vi "BStAT_(Doubles) Update.vi"() -> ()   [LabVIEW 2013]
uses:
  <vilib>/vision/Image Controls.llb/IMAQ Image.ctl
  <vilib>/Utility/file.llb/Read From Spreadsheet File (string).vi
  <vilib>/Utility/file.llb/Read From Spreadsheet File (I64).vi
panel:
  in  "fast rewind":bool
  out "refnum of data save file":refnum<file>
  in  "START":bool
  out "frames to write":i64[][](array[numeric])
  in  "Data file":path caption="Data"
  in  "playback speed":dbl(slide)=1.0 min=0.25 max=1.5 step=0.25 scale=0.25..1.5
  in  "Main tab":enum32{"Coding", "Display"}(tab)
  in  "9 6":bool
  in  "10 6":bool
  in  "9 5":bool
  in  "10 5":bool
  in  "10 3":bool
  in  "9 3":bool
  in  "10 4":bool
  in  "9 4":bool
  in  "9 2":bool
  in  "10 2":bool
  in  "10":bool
  in  "9":bool
  in  "1 6":bool
  in  "2 6":bool
  in  "3 6":bool
  in  "4 6":bool
  in  "5 6":bool
  in  "6 6":bool
  in  "7 6":bool
  in  "8 6":bool
  in  "1 5":bool
  in  "2 5":bool
  in  "3 5":bool
  in  "4 5":bool
  in  "5 5":bool
  in  "6 5":bool
  in  "7 5":bool
  in  "8 5":bool
  in  "8 3":bool
  in  "7 3":bool
  in  "6 3":bool
  in  "5 3":bool
  in  "4 3":bool
  in  "3 3":bool
  in  "2 3":bool
  in  "1 3":bool
  in  "8 4":bool
  in  "7 4":bool
  in  "6 4":bool
  in  "5 4":bool
  in  "4 4":bool
  in  "3 4":bool
  in  "2 4":bool
  in  "1 4":bool
  in  "1 2":bool
  in  "2 2":bool
  in  "3 2":bool
  in  "4 2":bool
  in  "5 2":bool
  in  "6 2":bool
  in  "7 2":bool
  in  "8 2":bool
  in  "5":bool
  in  "6":bool
  in  "7":bool
  in  "8":bool
  in  "1":bool
  in  "2":bool
  in  "3":bool
  in  "4":bool
  in  "Player 3":bool
  in  "Player 4":bool
  in  "MCL 3":bool
  in  "BCL 3":bool
  in  "TCL 3":bool
  in  "TCR 2":bool
  in  "MCR 2":bool
  in  "BCR 2":bool
  in  "TCR 3":bool
  in  "MCR  3":bool
  in  "BCR 3":bool
  in  "MCL 2":bool
  in  "BCL 2":bool
  in  "TCL 2":bool
  in  "Player 2":bool
  in  "Player 1":bool
  in  "TC 3":bool
  in  "TR 3":bool
  in  "ML 3":bool
  in  "MC 3":bool
  in  "MR  3":bool
  in  "BC 3":bool
  in  "BL 3":bool
  in  "BR 3":bool
  in  "TL 3":bool
  in  "TC 2":bool
  in  "TR 2":bool
  in  "ML 2":bool
  in  "MC 2":bool
  in  "MR  2":bool
  in  "BC 2":bool
  in  "BL 2":bool
  in  "BR 2":bool
  in  "TL 2":bool
  in  "Name 4":string
  in  "Name 3":string
  in  "Name 2":string
  in  "Name 1":string
  in  "5 7":bool
  in  "S3":bool
  in  "S4":bool
  in  "Switch position":bool
  in  "Link Errors":bool
  in  "E2":bool
  in  "E1":bool
  in  "W2":bool
  in  "W1":bool
  in  "P2":i32
  in  "P1":i32
  in  "S1":bool
  in  "S2":bool
  in  "1 7":bool
  in  "2 7":bool
  in  "3 7":bool
  in  "4 7":bool
  in  "Code lag(s)":dbl=1.0 min=0.0 max=5.0 step=0.5 format="%#.1g"
  in  "Pause lag(s)":dbl=1.0 min=0.0 max=2.0 step=0.5 format="%#.1g"
  in  "Pause lag on":bool
  in  "Display tab":enum32{"Edit ", "Data Display", "Momentum"}(tab)
  in  "player4":bool
  in  "player3":bool
  in  "player1":bool
  in  "player2":bool
  in  "Team 1":bool
  in  "Team 2":bool
  in  "service4":bool
  in  "service3":bool
  in  "5 8":bool
  in  "1 9":bool
  in  "service2":bool
  in  "service1":bool
  in  "2 9":bool
  in  "3 8":bool
  in  "4 8":bool
  in  "Blk def":bool
  in  "clear def":bool
  in  "lob":bool
  in  "clear":bool
  in  "drive":bool
  in  "smash":bool
  in  "Dr def":bool
  in  "Hf smash":bool
  in  "drop":bool
  in  "net":bool
  in  "FH 2":bool
  in  "BH 2":bool
  in  "ST":bool
  in  "CR 2":bool
  in  "OH 2":bool
  in  "BCR":bool
  in  "MCR":bool
  in  "TCR":bool
  in  "TCL":bool
  in  "BCL":bool
  in  "MCL":bool
  in  "TL":bool
  in  "BR":bool
  in  "BL":bool
  in  "BC":bool
  in  "MR":bool
  in  "MC":bool
  in  "ML":bool
  in  "TR":bool
  in  "TC":bool
  in  "REPORT":bool
  out "Video files to write":string[](array[string])
  in  "Video compress":bool=TRUE
  in  "Abort":bool
  in  "Write file":bool
  in  "Delete":bool[](array[boolean])
  out "Writing":u32(slide) scale=0.0..51.0
  in  "File name":string
  in  "Add to lib":bool
  in  "Video to write":path caption="Folder"
  in  "Examine code":bool
  in  "Update":bool
  in  "Reset":bool
  out "Code number display":i32
  in  "Next":bool
  in  "Previous":bool
  in  "after":u8(slide)=2 scale=0.0..5.0
  in  "before":u8(slide)=2
  in  "point 2":bool
  in  "error":bool
  in  "winner":bool
  in  "point 1":bool
  in  "Extract data":bool
  in  "Upload edited video":bool
  in  "To make white":enum32{""}(tab)
  out "player1 2":string[](array[string])=["0", "0", "0", "0", "0", "0", "0", "0", "0", "0"]
  out "player2 2":string[](array[string])=["0", "0", "0", "0", "0", "0", "0", "0", "0", "0"]
  out "p2 23":string
  out "p2 22":string
  out "p2 21":string
  out "p2 20":string
  out "p2 19":string
  out "p2 18":string
  out "p1 15":string
  out "p1 14":string
  out "p1 13":string
  out "p1 12":string
  out "p1 11":string
  out "p1 10":string
  out "p2 17":string
  out "p2 16":string
  out "p2 11":string
  out "p2 10":string
  out "p2 9":string
  out "p2 14":string
  out "p2 13":string
  out "p2 12":string
  out "p2 15":string
  out "p1 5":string
  out "p1 7":string
  out "p1 6":string
  out "p1 4":string
  out "p1 1":string
  out "p1 3":string
  out "p1 2":string
  out "p1 8":string
  out "p1 9":string
  out "Player 5":string[](array[string])=["Fore hand", "Back hand", "Over head", "", "Straight", "Cross", "", "Smash", "Half smash", "DRIVE DEF", "BLOCK DEF", "CLEAR DEF", "Drive/Tap", "Lob", "Drop", "Clear", "Net"]
  out "Player 6":string[](array[string])=["Fore hand", "Back hand", "Over head", "", "Straight", "Cross", "", "Smash", "Half smash", "DRIVE DEF", "BLOCK DEF", "CLEAR DEF", "Drive/Tap", "Lob", "Drop", "Clear", "Net"]
  out "player1_2":string[](array[string])=["0", "0", "0", "", "0", "0"]
  out "W2/E2":string[](array[string])=["0", "0"]
  out "Player 2_2":string[](array[string])=["Fore hand", "Back hand", "Over head", "", "Strainght", "Cross", "", "Lob", "Clear", "Drive", "Smash", "Defence", "Chop", "Drop", "Net"]
  out "W/E2":string[](array[string])=["Fore hand", "Back hand", "Over head", "", "Strainght", "Cross", "", "Lob", "Clear", "Drive", "Smash", "Defence", "Chop", "Drop", "Net"]
  out "player2_2":string[](array[string])=["0", "0", "0", "", "0", "0"]
  out "W1/E1":string[](array[string])=["0", "0"]
  out "Player 1_2":string[](array[string])=["Fore hand", "Back hand", "Over head", "", "Strainght", "Cross", "", "Lob", "Clear", "Drive", "Smash", "Defence", "Chop", "Drop", "Net"]
  out "W/E1":string[](array[string])=["Fore hand", "Back hand", "Over head", "", "Strainght", "Cross", "", "Lob", "Clear", "Drive", "Smash", "Defence", "Chop", "Drop", "Net"]
  out "P2graph":cluster{dbl[], "array":dbl[]}(graph)={[0.0, nan, 0.0, nan, 0.0, nan, 0.0, nan, 0.0, nan, 0.0, nan, 0.0, nan, 0.0, nan, 0.0], "array"=[1.0, 2.0, 3.0, 4.0, 5.0, 6.0, 7.0, 8.0, 9.0, 10.0, 11.0, 12.0, 13.0, 14.0, 15.0, 16.0, 17.0]}
  out "P1graph":cluster{dbl[], "array":dbl[]}(graph)={[0.0, nan, 0.0, nan, 0.0, nan, 0.0, nan, 0.0, nan, 0.0, nan, 0.0, nan, 0.0, nan, 0.0], "array"=[1.0, 2.0, 3.0, 4.0, 5.0, 6.0, 7.0, 8.0, 9.0, 10.0, 11.0, 12.0, 13.0, 14.0, 15.0, 16.0, 17.0]}
  in  "save2":string
  in  "save1":string
  in  "save2 3":bool
  in  "save1 3":bool
  in  "Compare":bool
  in  "2 8":string(combo)="1"
  in  "1 8":string(combo)="1"
  in  "display\nselection":string(combo)="1"
  in  "Percentage":bool
  in  "to make white 2":enum32{""}(tab)
  out "Shortest rally length(sec)":dbl format="%#_3g"
  out "Longest rally length(sec)":dbl format="%#_3g"
  out "Score":dbl[](array[numeric])
  out "Average rally length(sec)":dbl format="%#_3g"
  out "Rally length(sec)":dbl format="%#_3g"
  out "momentum graph":cluster{dbl[], dbl[]}[](graph)
  in  "Code number":i32 min=0 max=28
  in  "Load video":bool
  in  "Play":bool
  out "ful video frames":i64[](array[numeric])
  out "playback speed":dbl
  out "Number of Frames":u32
  out "framesPerSecond":u32
  out "Last Edit":bool[](array[boolean])
  out "frames 2 play":i64[](array[numeric])
  in  "stop":bool
  out "Video Frame":u32
  out "save1 2":i32[][](array[numeric])
  out "save1_data":dbl[][](array[numeric])
  out "save2 2":i32[][](array[numeric])
  out "save2_data":dbl[][](array[numeric])
  out "game":i32[][](array[numeric])
  out "comp_p1":dbl[](array[numeric])
  out "comp_p2":dbl[](array[numeric])
  out "comp_p2 2":dbl[](array[numeric])
  out "comp_p1 2":dbl[](array[numeric])
  out "Score 2":i64[][](array[numeric])
  out "frame data":i64[][](array[numeric])
  out "coded data":i64[][](array[numeric])
  out "edited\nevents":i64[][](array[numeric])
  out "edited to play":i64[](array[numeric])
  out "frames edited":i64[](array[numeric])
  out "service frames":i64[](array[numeric])
  out "point frames":i64[](array[numeric])
  out "p1y":dbl[](array[numeric])
  out "p2y":dbl[](array[numeric])
  in  "fast forward":bool
  in  "Pause":bool
  out "coding":i64[][](array[numeric])
  out "FH":bool[](array[boolean])
  out "BH":bool[](array[boolean])
  out "OH":bool[](array[boolean])
  out "P1 position":bool
  out "P2 position":bool
  in  "Progress...":u32(slide) min=400 max=47374 scale=-1.1..47174.0
  in  "Video file":path caption="Video"
  out "task":i32(slide) scale=0.0..300.0
  out "Video":T1(plugin-control)
  # "Strategic Analysis Tool for Badminton"
  # "© 2012 National Sports Institute of Malaysia All Rights Reserved"
  # "Position"
  # "Rally start"
  # "Rally end"
  # "Forehand"
  # "Backhand"
  # "Overhead"
  # "Straight"
  # "Cross"
  # "Straight"
  # "Cross"
  # "Straight"
  # "Cross"
  # "Smash"
  # "Half Smash"
  # "DRIVE Defence"
  # "BLOCK Defence"
  # "CLEAR Defence"
  # "Drive/Tap"
  # "Lob"
  # "Drop"
  # "Clear"
  # "Net"
  # "Switch sides"
  # "Player"
  # "Team"
  # "Rally start"
  # "Shots"
  # "Position"
  # "Playback interval (s)"
  # "Rally end"
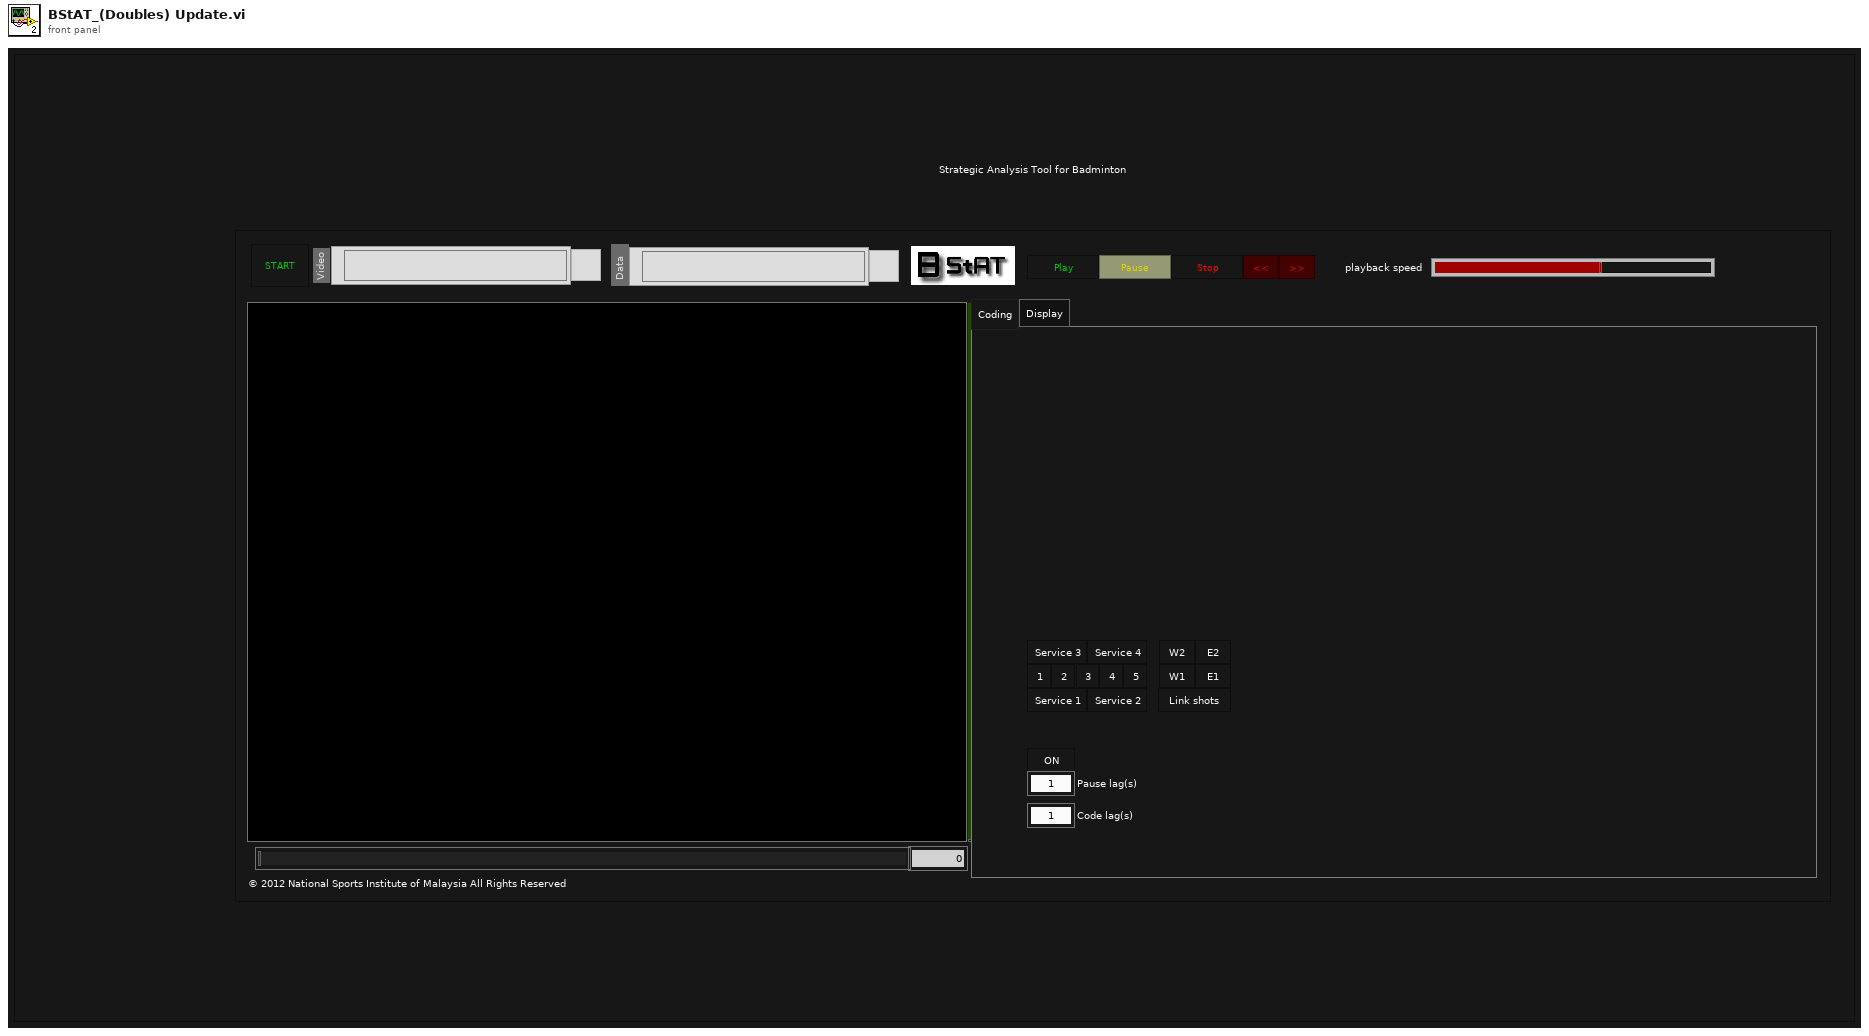
[diagram p1: front panel]
types:
  T1 = typedef "IMAQ Image.ctl" = refnum<image>
  T2 = enum32{"Coding", "Edit video", "Examine coding", "Display", "Update coding", "Edit coding"}
  T3 = enum16{"open", "replace", "create", "open or create", "replace or create", "replace or create with confirmation"}
  T4 = enum8{"Enabled", "Disabled", "Disabled and Grayed Out"}
  T5 = typedef "Image Type" = u32
  T6 = typedef "AviRefnum.ctl" = refnum<k1>
  T7 = cluster{"width":u32, "height":u32, "framesPerSecond":u32, "compressionFilter":string, "hasData":bool}
  T8 = typedef "LVPositionTypeDef.ctl" = cluster{"Left":i32, "Top":i32}
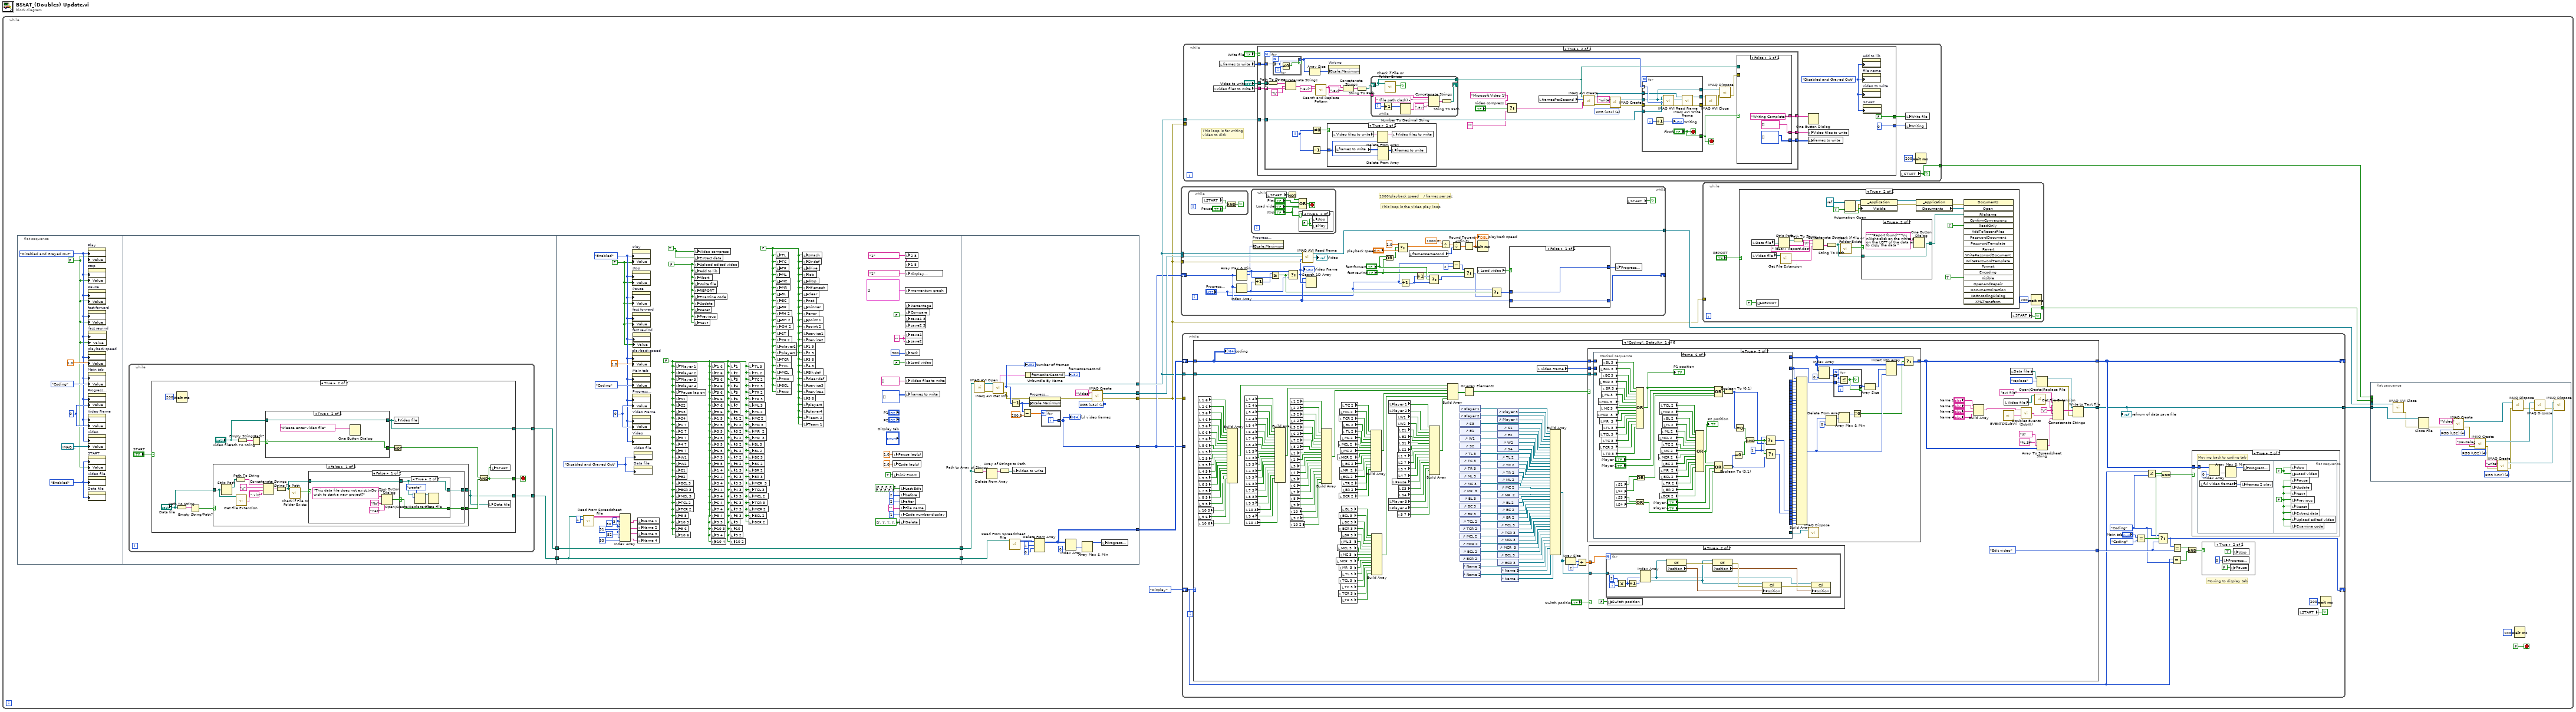
[diagram p0: block diagram]
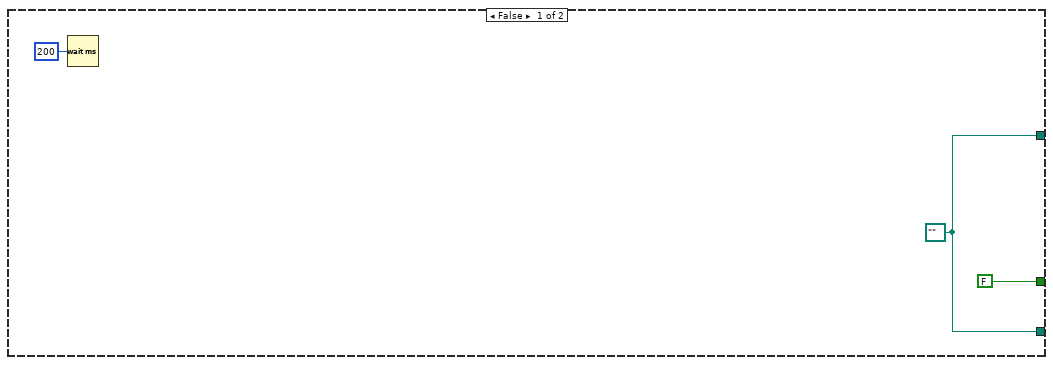
[diagram p2: hidden frame]
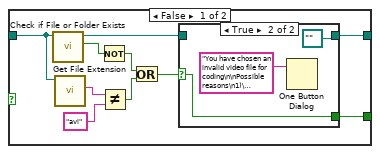
[diagram p3: hidden frame]
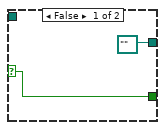
[diagram p5: hidden frame]
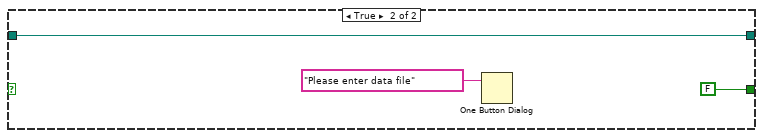
[diagram p7: hidden frame]
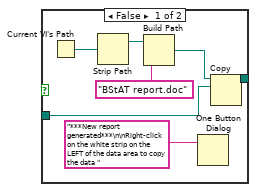
[diagram p9: hidden frame]
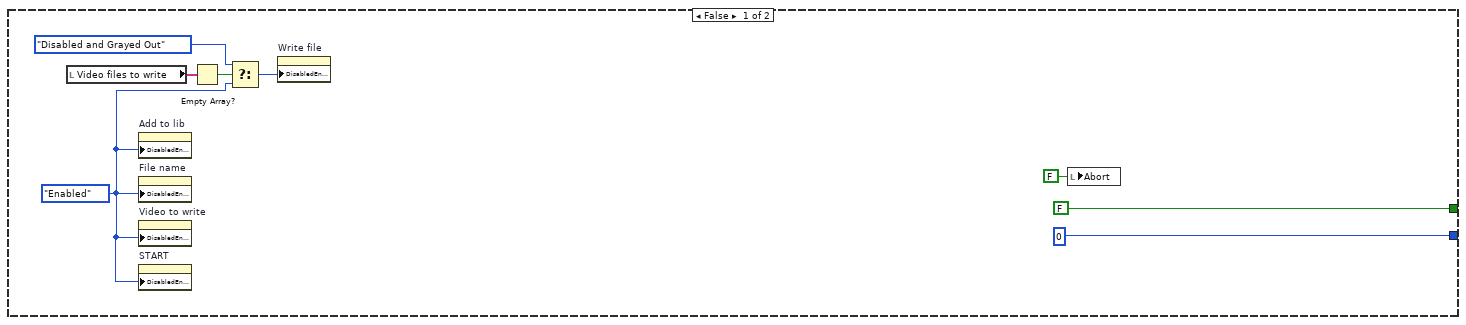
[diagram p10: hidden frame]
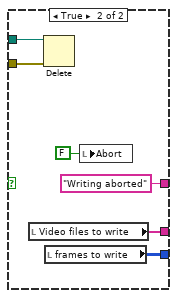
[diagram p11: hidden frame]
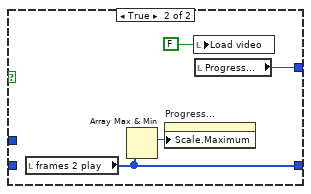
[diagram p14: hidden frame]
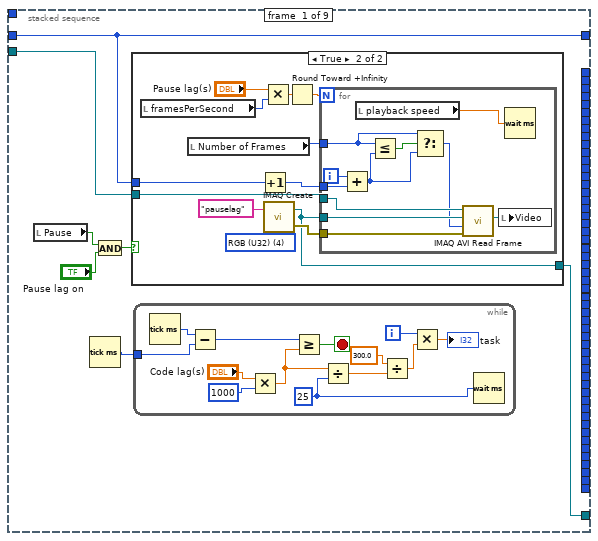
[diagram p19: hidden frame]
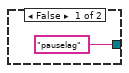
[diagram p20: hidden frame]
diagram:
  n1 = while {
    stop <- FALSE stop-if-true
    n2 = flat-sequence {
      tunnel: [w42] -> w15
      tunnel: [w43] -> w16
      tunnel: w16 -> [w152]
      tunnel: w15 -> [w133]
      tunnel: [w133] -> w14
      tunnel: [w152] -> w13
      tunnel: w14 -> [w174]
      tunnel: w13 -> [w157]
      tunnel: [w173] -> w11
      tunnel: [w156] -> w10
      tunnel: [w155] -> w9
      tunnel: [w154] -> w1
      tunnel: [w153] -> w8
      frame #0 {
        w37 = T4."Enabled" ("Disabled")
        w39 = u32 0 ("Progress...")
        w35 = FALSE ("START")
        w36 = T4."Disabled and Grayed Out" ("Disabled")
        n3 = property on="Play" class="Bool (strict)"("DisabledEnum"=w36, "Value"=w35) -> ()  [unwired: 2 in, 2 out]
        n4 = property on="stop" class="Bool (strict)"("DisabledEnum"=w36, "Value"=w35) -> ()  [unwired: 2 in, 2 out]
        n5 = property on="Pause" class="Bool (strict)"("DisabledEnum"=w36, "Value"=w35) -> ()  [unwired: 2 in, 2 out]
        n6 = property on="fast forward" class="Bool (strict)"("DisabledEnum"=w36, "Value"=w35) -> ()  [unwired: 2 in, 2 out]
        n7 = property on="playback speed" class="Slide (strict)"("DisabledEnum"=w36, "Value"=1.0 ("playback speed")) -> ()  [unwired: 2 in, 2 out]
        n8 = property on="Main tab" class="TabCtl (strict)"("DisabledEnum"=w36, "Value"=enum32{"Coding", "Display"}."Coding" ("Main tab")) -> ()  [unwired: 2 in, 2 out]
        n9 = property on="Progress..." class="Slide (strict)"("DisabledEnum"=w36, "Value"=w39) -> ()  [unwired: 2 in, 2 out]
        n10 = property on="Video Frame" class="DigNum (strict)"("DisabledEnum"=w36, "Value"=w39) -> ()  [unwired: 2 in, 2 out]
        n11 = property on="Video" class="ImageControl"("DisabledEnum"=w36, "Value"=T1 refnum ("Video")) -> ()  [unwired: 2 in, 2 out]
        n12 = property on="START" class="Bool (strict)"("DisabledEnum"=w37, "Value"=w35) -> ()  [unwired: 2 in, 2 out]
        n13 = property on="Video file" class="Path"("DisabledEnum"=w37) -> ()  [unwired: 2 in, 2 out]
        n14 = property on="Data file" class="Path"("DisabledEnum"=w37) -> ()  [unwired: 2 in, 2 out]
        n15 = property on="fast rewind" class="Bool (strict)"("DisabledEnum"=w36, "Value"=w35) -> ()  [unwired: 2 in, 2 out]
      }
      frame #1 {
        n16 = while {
          tunnel: [w45] -> w43
          tunnel: [w44] -> w42
          stop <- w46 stop-if-true
          n17 = case shown="True" "START" {
            tunnel: [FALSE w51] -> w46
            tunnel: [w48 w54] -> w45
            tunnel: [w48 w53] -> w44
            frame False {
              w48 = path "" ("dup path")
              n18 = Wait (ms)(milliseconds to wait=u32 200) -> ()  [unwired: 1 out]
            }
            frame True {
              n19 = Path To String(path="Data file") -> (string=w63:string)
              n20 = Wait (ms)(milliseconds to wait=u32 200) -> ()  [unwired: 1 out]
              n21 = Empty String/Path?(string/path=w63) -> (empty?=w62:bool)
              n22 = case shown="False" w62 {
                tunnel: "Data file" -> [w84 w109]
                tunnel: [w83 FALSE] -> w60
                tunnel: [w82 w109] -> w53
                frame False {
                  n23 = Strip Path(path=w84) -> (stripped path=w89:path)  [unwired: 1 out]
                  n24 = Path To String(path=w89) -> (string=w88:string)
                  n25 = call <vilib>:"Get File Extension.vi"("file"=w84) -> ("filename without extension"=w91:string)  [unwired: 7 in, 3 out]
                  n26 = Concatenate Strings(w88, "\\" ("string"), w91, ".xls" ("string")) -> (w90:string)
                  n27 = String To Path(string=w90) -> (path=w85:path)
                  n28 = call <vilib>:"Check if File or Folder Exists.vi"("path"=w85) -> ("file or folder exists?"=w86:bool)  [unwired: 8 in, 2 out]
                  n29 = case shown="False" w86 {
                    selector: w86 -> [_ w108]
                    tunnel: w85 -> [w95 w107]
                    tunnel: [w94 w108] -> w83
                    tunnel: [w93 w107] -> w82
                    frame False {
                      n30 = Two Button Dialog(message="This data file does not exist.\nDo you wish to start a new project?", 1:"No" ("F button name (\"Cancel\")"), 2:"Yes" ("T button name (\"OK\")")) -> (T button?=w96:bool)
                      n31 = case shown="True" w96 {
                        selector: w96 -> [w101 w103]
                        tunnel: w95 -> [_ w102]
                        tunnel: [w101 w103] -> w94
                        tunnel: [path "" ("dup path") w102] -> w93
                        frame False {
                        }
                        frame True {
                          n32 = Open/Create/Replace File(file path (use dialog)=w102, operation (0:open)=T3."create") -> (refnum out=w104:refnum<file>, error out=w106:errorcluster)  [unwired: 4 in, 1 out]
                          n33 = Close File(refnum=w104, error in=w106) -> ()  [unwired: 2 out]
                        }
                      }
                    }
                    frame True {
                    }
                  }
                }
                frame True {
                  n34 = One Button Dialog(message="Please enter data file") -> ()  [unwired: 1 in, 1 out]
                }
              }
              n35 = Path To String(path="Video file") -> (string=w58:string)
              n36 = Empty String/Path?(string/path=w58) -> (empty?=w57:bool)
              n37 = case shown="True" w57 {
                selector: w57 -> [_ w81]
                tunnel: "Video file" -> [w68 w79]
                tunnel: [w65 w79] -> w54
                tunnel: [w64 w81] -> w55
                frame False {
                  n38 = call <vilib>:"Check if File or Folder Exists.vi"("path"=w68) -> ("file or folder exists?"=w72:bool, "dup path"=w66:path)  [unwired: 8 in, 1 out]
                  n39 = call <vilib>:"Get File Extension.vi"("file"=w68) -> ("lowercase file extension"=w69:string)  [unwired: 7 in, 3 out]
                  n40 = Not(x=w72) -> (.not. x?=w73:bool)
                  n41 = Not Equal?(x=w69, y="avi" ("lowercase file extension")) -> (x != y?=w71:bool)
                  n42 = Or(x=w73, y=w71) -> (x .or. y?=w67:bool)
                  n43 = case shown="True" w67 {
                    selector: w67 -> [w74 w76]
                    tunnel: w66 -> [w75 _]
                    tunnel: [w75 path "" ("dup path")] -> w65
                    tunnel: [w74 w76] -> w64
                    frame False {
                    }
                    frame True {
                      n44 = One Button Dialog(message="You have chosen an invalid video file for coding\n\nPossible reasons\n1)\tChosen video file format was not AVI\n2)\tChosen video file does not exist") -> ()  [unwired: 1 in, 1 out]
                    }
                  }
                }
                frame True {
                  n45 = One Button Dialog(message="Please enter video file") -> ()  [unwired: 1 in, 1 out]
                }
              }
              n46 = Not(x=w55) -> (.not. x?=w59:bool)
              n47 = local write "Video file"(w54) -> ()
              n48 = And(x=w59, y=w60) -> (x .and. y?=w51:bool)
              n49 = local write "Data file"(w53) -> ()
              n50 = local write "START"(w51) -> ()
            }
          }
        }
      }
      frame #2 {
        w130 = 3 ("index (row)")
        w138 = "" ("save2")
        w139 = "1" ("2 8")
        w142 = FALSE ("4 6")
        w121 = FALSE ("4 6")
        w147 = FALSE ("4 6")
        w120 = FALSE ("4 6")
        w146 = TRUE ("Extract data")
        w148 = T4."Disabled and Grayed Out" ("Disabled")
        w151 = u32 0 ("Progress...")
        w112 = FALSE ("START")
        w113 = T4."Enabled" ("Disabled")
        n51 = call-poly <vilib>:"Read From Spreadsheet File.vi"("number of rows (all:-1)"=4, "file path (dialog if empty)"=w133) -> ("all rows"=w131:string[][])  [unwired: 5 in, 4 out]
        n52 = Index Array(array=w131, index (row) #1=w130, index (col) #1=50 ("disabled index (col)"), index (row) #2=w130, index (col) #2=51 ("disabled index (col)"), index (row) #3=w130, index (col) #3=52 ("disabled index (col)"), index (row) #4=w130, index (col) #4=53 ("disabled index (col)")) -> (element #1=w122:string, element #2=w125:string, element #3=w124:string, element #4=w123:string)
        n53 = property on="Play" class="Bool (strict)"("DisabledEnum"=w113, "Value"=w112) -> ()  [unwired: 2 in, 2 out]
        n54 = property on="stop" class="Bool (strict)"("DisabledEnum"=w113, "Value"=w112) -> ()  [unwired: 2 in, 2 out]
        n55 = property on="Pause" class="Bool (strict)"("DisabledEnum"=w113, "Value"=w112) -> ()  [unwired: 2 in, 2 out]
        n56 = property on="fast forward" class="Bool (strict)"("DisabledEnum"=w113, "Value"=w112) -> ()  [unwired: 2 in, 2 out]
        n57 = property on="playback speed" class="Slide (strict)"("DisabledEnum"=w113, "Value"=1.0 ("playback speed")) -> ()  [unwired: 2 in, 2 out]
        n58 = property on="Main tab" class="TabCtl (strict)"("DisabledEnum"=w113, "Value"=enum32{"Coding", "Display"}."Coding" ("Main tab")) -> ()  [unwired: 2 in, 2 out]
        n59 = property on="Progress..." class="Slide (strict)"("DisabledEnum"=w113, "Value"=w151) -> ()  [unwired: 2 in, 2 out]
        n60 = property on="Video Frame" class="DigNum (strict)"("DisabledEnum"=w113, "Value"=w151) -> ()  [unwired: 2 in, 2 out]
        n61 = property on="Video" class="ImageControl"("DisabledEnum"=w113) -> ()  [unwired: 2 in, 2 out]
        n62 = property on="fast rewind" class="Bool (strict)"("DisabledEnum"=w113, "Value"=w112) -> ()  [unwired: 2 in, 2 out]
        n63 = property on="Video file" class="Path"("DisabledEnum"=w148) -> ()  [unwired: 2 in, 2 out]
        n64 = property on="Data file" class="Path"("DisabledEnum"=w148) -> ()  [unwired: 2 in, 2 out]
        n65 = local write "Name 1"(w122) -> ()
        n66 = local write "Name 2"(w125) -> ()
        n67 = local write "Name 3"(w124) -> ()
        n68 = local write "Name 4"(w123) -> ()
        n69 = local write "Player 1"(w121) -> ()
        n70 = local write "Player 2"(w121) -> ()
        n71 = local write "Player 3"(w121) -> ()
        n72 = local write "Player 4"(w121) -> ()
        n73 = local write "Pause lag on"(w121) -> ()
        n74 = local write "S1"(w121) -> ()
        n75 = local write "S2"(w121) -> ()
        n76 = local write "S3"(w121) -> ()
        n77 = local write "S4"(w121) -> ()
        n78 = local write "1 7"(w121) -> ()
        n79 = local write "2 7"(w121) -> ()
        n80 = local write "3 7"(w121) -> ()
        n81 = local write "4 7"(w121) -> ()
        n82 = local write "5 7"(w121) -> ()
        n83 = local write "W1"(w121) -> ()
        n84 = local write "W2"(w121) -> ()
        n85 = local write "E1"(w121) -> ()
        n86 = local write "E2"(w121) -> ()
        n87 = local write "BCL 3"(w121) -> ()
        n88 = local write "BCR 3"(w121) -> ()
        n89 = local write "MCL 3"(w121) -> ()
        n90 = local write "TCL 2"(w121) -> ()
        n91 = local write "TCR 2"(w121) -> ()
        n92 = local write "9 5"(w121) -> ()
        n93 = local write "10 5"(w121) -> ()
        n94 = local write "9 6"(w121) -> ()
        n95 = local write "10 6"(w121) -> ()
        n96 = local write "Video compress"(w146) -> ()
        n97 = local write "Extract data"(w146) -> ()
        n98 = local write "Upload edited video"(w147) -> ()
        n99 = local write "Add to lib"(w147) -> ()
        n100 = local write "Abort"(w147) -> ()
        n101 = local write "Write file"(w147) -> ()
        n102 = local write "REPORT"(w147) -> ()
        n103 = local write "Examine code"(w147) -> ()
        n104 = local write "Update"(w147) -> ()
        n105 = local write "Reset"(w147) -> ()
        n106 = local write "Previous"(w147) -> ()
        n107 = local write "Next"(w147) -> ()
        n108 = local write "1 6"(w121) -> ()
        n109 = local write "2 6"(w121) -> ()
        n110 = local write "3 6"(w121) -> ()
        n111 = local write "4 6"(w121) -> ()
        n112 = local write "5 6"(w121) -> ()
        n113 = local write "6 6"(w121) -> ()
        n114 = local write "7 6"(w121) -> ()
        n115 = local write "8 6"(w121) -> ()
        n116 = local write "1 5"(w121) -> ()
        n117 = local write "2 5"(w121) -> ()
        n118 = local write "3 5"(w121) -> ()
        n119 = local write "4 5"(w121) -> ()
        n120 = local write "5 5"(w121) -> ()
        n121 = local write "6 5"(w121) -> ()
        n122 = local write "7 5"(w121) -> ()
        n123 = local write "8 5"(w121) -> ()
        n124 = local write "1 4"(w121) -> ()
        n125 = local write "2 4"(w121) -> ()
        n126 = local write "3 4"(w121) -> ()
        n127 = local write "4 4"(w121) -> ()
        n128 = local write "5 4"(w121) -> ()
        n129 = local write "6 4"(w121) -> ()
        n130 = local write "7 4"(w121) -> ()
        n131 = local write "8 4"(w121) -> ()
        n132 = local write "9 3"(w121) -> ()
        n133 = local write "10 3"(w121) -> ()
        n134 = local write "9 4"(w121) -> ()
        n135 = local write "10 4"(w121) -> ()
        n136 = local write "1"(w121) -> ()
        n137 = local write "2"(w121) -> ()
        n138 = local write "3"(w121) -> ()
        n139 = local write "4"(w121) -> ()
        n140 = local write "5"(w121) -> ()
        n141 = local write "6"(w121) -> ()
        n142 = local write "7"(w121) -> ()
        n143 = local write "8"(w121) -> ()
        n144 = local write "1 2"(w121) -> ()
        n145 = local write "2 2"(w121) -> ()
        n146 = local write "3 2"(w121) -> ()
        n147 = local write "4 2"(w121) -> ()
        n148 = local write "5 2"(w121) -> ()
        n149 = local write "6 2"(w121) -> ()
        n150 = local write "7 2"(w121) -> ()
        n151 = local write "8 2"(w121) -> ()
        n152 = local write "1 3"(w121) -> ()
        n153 = local write "2 3"(w121) -> ()
        n154 = local write "3 3"(w121) -> ()
        n155 = local write "4 3"(w121) -> ()
        n156 = local write "5 3"(w121) -> ()
        n157 = local write "6 3"(w121) -> ()
        n158 = local write "7 3"(w121) -> ()
        n159 = local write "8 3"(w121) -> ()
        n160 = local write "9"(w121) -> ()
        n161 = local write "10"(w121) -> ()
        n162 = local write "9 2"(w121) -> ()
        n163 = local write "10 2"(w121) -> ()
        n164 = local write "TL 3"(w121) -> ()
        n165 = local write "TL 2"(w121) -> ()
        n166 = local write "TC 2"(w121) -> ()
        n167 = local write "TC 3"(w121) -> ()
        n168 = local write "TR 2"(w121) -> ()
        n169 = local write "TR 3"(w121) -> ()
        n170 = local write "ML 3"(w121) -> ()
        n171 = local write "ML 2"(w121) -> ()
        n172 = local write "MC 2"(w121) -> ()
        n173 = local write "MC 3"(w121) -> ()
        n174 = local write "MR  2"(w121) -> ()
        n175 = local write "MR  3"(w121) -> ()
        n176 = local write "BL 3"(w121) -> ()
        n177 = local write "BL 2"(w121) -> ()
        n178 = local write "BC 3"(w121) -> ()
        n179 = local write "BC 2"(w121) -> ()
        n180 = local write "BR 2"(w121) -> ()
        n181 = local write "BR 3"(w121) -> ()
        n182 = local write "MCR  3"(w121) -> ()
        n183 = local write "TCL 3"(w121) -> ()
        n184 = local write "MCL 2"(w121) -> ()
        n185 = local write "TCR 3"(w121) -> ()
        n186 = local write "MCR 2"(w121) -> ()
        n187 = local write "BCL 2"(w121) -> ()
        n188 = local write "BCR 2"(w121) -> ()
        n189 = local write "TL"(w120) -> ()
        n190 = local write "TC"(w120) -> ()
        n191 = local write "TR"(w120) -> ()
        n192 = local write "ML"(w120) -> ()
        n193 = local write "MC"(w120) -> ()
        n194 = local write "MR"(w120) -> ()
        n195 = local write "BL"(w120) -> ()
        n196 = local write "BC"(w120) -> ()
        n197 = local write "BR"(w120) -> ()
        n198 = local write "FH 2"(w120) -> ()
        n199 = local write "BH 2"(w120) -> ()
        n200 = local write "OH 2"(w120) -> ()
        n201 = local write "ST"(w120) -> ()
        n202 = local write "CR 2"(w120) -> ()
        n203 = local write "player1"(w120) -> ()
        n204 = local write "player2"(w120) -> ()
        n205 = local write "TCR"(w120) -> ()
        n206 = local write "TCL"(w120) -> ()
        n207 = local write "MCL"(w120) -> ()
        n208 = local write "MCR"(w120) -> ()
        n209 = local write "BCL"(w120) -> ()
        n210 = local write "BCR"(w120) -> ()
        n211 = local write "smash"(w120) -> ()
        n212 = local write "Dr def"(w120) -> ()
        n213 = local write "drive"(w120) -> ()
        n214 = local write "lob"(w120) -> ()
        n215 = local write "drop"(w120) -> ()
        n216 = local write "Hf smash"(w120) -> ()
        n217 = local write "clear"(w120) -> ()
        n218 = local write "net"(w120) -> ()
        n219 = local write "winner"(w120) -> ()
        n220 = local write "error"(w120) -> ()
        n221 = local write "point 1"(w120) -> ()
        n222 = local write "point 2"(w120) -> ()
        n223 = local write "service1"(w120) -> ()
        n224 = local write "service2"(w120) -> ()
        n225 = local write "1 9"(w120) -> ()
        n226 = local write "2 9"(w120) -> ()
        n227 = local write "3 8"(w120) -> ()
        n228 = local write "4 8"(w120) -> ()
        n229 = local write "Blk def"(w120) -> ()
        n230 = local write "clear def"(w120) -> ()
        n231 = local write "service3"(w120) -> ()
        n232 = local write "service4"(w120) -> ()
        n233 = local write "5 8"(w120) -> ()
        n234 = local write "player3"(w120) -> ()
        n235 = local write "player4"(w120) -> ()
        n236 = local write "Team 2"(w120) -> ()
        n237 = local write "Team 1"(w120) -> ()
        n238 = local write "Pause lag(s)"(1.0 ("Pause lag(s)")) -> ()
        n239 = local write "Code lag(s)"(2.0 ("Code lag(s)")) -> ()
        n240 = local write "Link Errors"(TRUE ("Link Errors")) -> ()
        n241 = local write "Last Edit"(bool[] [FALSE, FALSE, FALSE, FALSE, FALSE, FALSE, FALSE, FALSE, FALSE, FALSE, FALSE, FALSE, FALSE, FALSE, FALSE, FALSE, FALSE, FALSE, FALSE, FALSE, FALSE, FALSE, FALSE, FALSE, FALSE, FALSE, FALSE, FALSE, FALSE, FALSE, FALSE, FALSE, FALSE, FALSE, FALSE, FALSE] ("Last Edit")) -> ()
        n242 = local write "before"(u8 2 ("before")) -> ()
        n243 = local write "after"(u8 2 ("after")) -> ()
        n244 = local write "File name"("" ("File name")) -> ()
        n245 = local write "Code number display"(1 ("Code number display")) -> ()
        n246 = local write "Delete"(bool[] [TRUE, TRUE, TRUE, TRUE, TRUE] ("Array 2")) -> ()
        n247 = local write "2 8"(w139) -> ()
        n248 = local write "1 8"(w139) -> ()
        n249 = local write "display\nselection"("1" ("display\nselection")) -> ()
        n250 = local write "momentum graph"(cluster{dbl[], dbl[]}[] [] ("momentum graph")) -> ()
        n251 = local write "Percentage"(w142) -> ()
        n252 = local write "Compare"(w142) -> ()
        n253 = local write "save1 3"(w142) -> ()
        n254 = local write "save2 3"(w142) -> ()
        n255 = local write "save1"(w138) -> ()
        n256 = local write "save2"(w138) -> ()
        n257 = local write "task"(300 ("task")) -> ()
        n258 = local write "Load video"(FALSE ("Pause")) -> ()
        n259 = local write "Video files to write"(string[] [] ("Video files to write")) -> ()
        n260 = local write "frames to write"(i64[][] [] ("to write")) -> ()
      }
      frame #3 {
        w159 = T5 4 items=["Grayscale (U8)", "Grayscale (I16)", "Grayscale (SGL)", "Complex (CSG)", "RGB (U32)", "HSL (U32)", "RGB (U64)"] ("Image Type")
        n261 = Path to Array of Strings(0:w157) -> (2:w170:string[])  [unwired: 1 out]
        n262 = call "IMAQ AVI Open"("AVI Path"=w157) -> ("error out"=w161:errorcluster, "Avi Refnum"=w160:T6)  [unwired: 9 in]
        n263 = Delete From Array(array=w170) -> (array with subset deleted=w171:string[])  [unwired: 2 in, 1 out]
        n264 = call "IMAQ AVI Get Info"("error in (no error)"=w161, "Avi Refnum"=w160) -> ("error out"=w163:errorcluster, "Number of Frames"=w166:u32, "Avi Refnum (duplicate)"=w156:T6, "Frame Data"=w162:T7)  [unwired: 5 in, 1 out]
        "Number of Frames" <- w166
        n265 = Array of Strings to Path(0:w171) -> (2:w172:path)  [unwired: 1 in]
        n266 = call-poly <vilib>:"Read From Spreadsheet File.vi"("file path (dialog if empty)"=w174) -> ("all rows"=w177:i64[][])  [unwired: 6 in, 4 out]
        n267 = Decrement(x=w166) -> (x-1=w169:u32)
        n268 = local write "Video to write"(w172) -> ()
        n269 = Subtract(x=w169, y=200.0) -> (x-y=w167:dbl)
        n270 = Unbundle By Name(w162) -> ("framesPerSecond"=→"framesPerSecond":u32)
        n271 = property on="Progress..." class="Slide (strict)"(error in=w163, "Scale.Maximum"=w169) -> (error out=w164:errorcluster)  [unwired: 1 in, 1 out]
        n272 = Delete From Array(array=w177, length=4, index (row)=0) -> (array with subset deleted=w173:i64[][])  [unwired: 1 in, 1 out]
        n273 = for {
          N: w167 -> [_]
          tunnel: [w181] -> w153 mode=indexing
          i -> [w181]
        }
        "ful video frames" <- w153
        n274 = Index Array(array=w173, index (col)=0 ("disabled index (col)")) -> (element=w179:i64[])  [unwired: 1 in]
        n275 = Array Max & Min(array=w179) -> (max value=w178:i64)  [unwired: 3 out]
        n276 = call "IMAQ Create"("Image Name"="Video", "Image Type"=w159, "error in (no error)"=w164) -> ("New Image"=w155:T1, "error out"=w154:errorcluster)  [unwired: 2 in]
        n277 = local write "Progress..."(w178) -> ()
      }
    }
    n278 = while {
      tunnel: w10 -> [w353]
      tunnel: w9 -> [w352]
      tunnel: w1 -> [w351]
      shift-right: [w345] -> _
      shift-left: w8 -> [w344]
      tunnel: [w329] -> w4
      stop <- w330 continue-if-true
      # "This loop is the video play loop"
      # "1000/playback speed    / frames per sec"
      n279 = while {
        stop <- w369 continue-if-true
        n280 = local read "START"() -> (w368:bool)
        n281 = And(x=w368, y="Pause") -> (x .and. y?=w369:bool)
      }
      n282 = Index Array(array=w344, index="Progress...") -> (element=w331:i64)
      n283 = Array Max & Min(array=w344) -> (max value=w349:i64, max index (indices)=w350:i32)  [unwired: 2 out]
      n284 = while {
        stop <- w358 stop-if-true
        n285 = local read "START"() -> (w355:bool)
        n286 = Not(x=w355) -> (.not. x?=w354:bool)
        n287 = Compound Arithmetic op=OR(w354, "Play", "Load video", "stop") -> (w358:bool)
        n288 = case shown="True" "stop" {
          frame False {
          }
          frame True {
            w360 = FALSE ("Play")
            n289 = local write "stop"(w360) -> ()
            n290 = local write "Play"(w360) -> ()
          }
        }
      }
      n291 = property on="Progress..." class="Slide (strict)"("Scale.Maximum"=w350) -> ()  [unwired: 2 in, 2 out]
      n292 = Increment(x=w331) -> (x+1=w332:i64)
      n293 = Greater Or Equal?(x=w332, y=w349) -> (x >= y?=w335:bool)
      n294 = Select(t=w349, s=w335, f=w331) -> (s? t:f=w346:i64)
      "Video Frame" <- w346
      n295 = call "IMAQ AVI Read Frame"("error in (no error)"=w351, "Frame Number"=w346, "Image"=w352, "Avi Refnum"=w353) -> ("Image Out"=→"Video":T1, "Avi Refnum (duplicate)"=w329:T6)  [unwired: 4 in, 2 out]
      n296 = Search 1D Array(1D array=w344, element=w346) -> ()  [unwired: 1 in, 1 out]
      n297 = Or(x="fast forward", y="fast rewind") -> (x .or. y?=w323:bool)
      n298 = Select(t=1.0, s=w323, f="playback speed") -> (s? t:f=w338:dbl)
      n299 = Increment(x="Progress...") -> (x+1=w325:u32)
      n300 = local read "framesPerSecond"() -> (w343:u32)
      n301 = Increment(x=w325) -> (x+1=w324:u32)
      n302 = Select(t=w324, s="fast forward", f=w325) -> (s? t:f=w327:u32)
      n303 = Divide(x=1000.0, y=w338) -> (x/y=w342:dbl)
      n304 = Subtract(x="Progress...", y=2) -> (x-y=w326:u32)
      n305 = Divide(x=w342, y=w343) -> (x/y=w340:dbl)
      n306 = Round Toward -Infinity(1:w340) -> (0:w339:dbl)
      "playback speed" <- w339
      n307 = Select(t=w326, s="fast rewind", f=w327) -> (s? t:f=w322:u32)
      n308 = Wait (ms)(milliseconds to wait=w339) -> ()  [unwired: 1 out]
      n309 = local read "Load video"() -> (w333:bool)
      n310 = Select(t="Progress...", s=w335, f=w322) -> (s? t:f=w334:u32)
      n311 = case shown="False" w333 {
        tunnel: w344 -> [w361 _]
        tunnel: w334 -> [w362 _]
        tunnel: [w362 w363] -> w348
        tunnel: [w361 w366] -> w345
        frame False {
        }
        frame True {
          n312 = local read "frames 2 play"() -> (w366:i64[])
          n313 = Array Max & Min(array=w366) -> (max index (indices)=w365:i32)  [unwired: 3 out]
          n314 = property on="Progress..." class="Slide (strict)"("Scale.Maximum"=w365) -> ()  [unwired: 2 in, 2 out]
          n315 = local write "Load video"(FALSE ("Play")) -> ()
          n316 = local read "Progress..."() -> (w363:u32)
        }
      }
      n317 = local write "Progress..."(w348) -> ()
      n318 = local read "START"() -> (w330:bool)
    }
    n319 = while {
      shift-right: [w379] -> _
      shift-left: T2."Display" ("Main tab") -> [w376]
      tunnel: w10 -> [w384]
      shift-right: [w372] -> _
      shift-left: w11 -> [w387]
      tunnel: w8 -> [_]
      tunnel: w1 -> [_]
      tunnel: [w370] -> w7
      stop <- w371 continue-if-true
      w375 = T2."Coding" ("Main tab")
      # "Moving to display tab"
      n320 = case shown="\"Coding\", Default" w376 {
        tunnel: w387 -> [w590 w1079 w1624 w1841 w1881 w1986]
        tunnel: [w511 w1079 w1624 w1841 w1881 w1972] -> w372
        tunnel: [T2."Edit video" ("Main tab") w1082 T2."Display" ("Main tab") T2."Edit coding" ("Main tab") w1882 T2."Edit video" ("Main tab")] -> w378
        tunnel: w384 -> [w523 _ _ _ _ _]
        tunnel: [w506 w1073 w1675 w1839 w1879 w1970] -> w370
        frame "Coding", Default {
          w517 = "\r"
          n321 = local read "1 6"() -> (w573:bool)
          n322 = local read "2 6"() -> (w574:bool)
          n323 = local read "3 6"() -> (w575:bool)
          n324 = local read "4 6"() -> (w576:bool)
          n325 = local read "5 6"() -> (w577:bool)
          n326 = local read "6 6"() -> (w578:bool)
          n327 = local read "7 6"() -> (w580:bool)
          n328 = local read "8 6"() -> (w579:bool)
          n329 = local read "1 5"() -> (w581:bool)
          n330 = local read "2 5"() -> (w582:bool)
          n331 = local read "3 5"() -> (w583:bool)
          n332 = local read "4 5"() -> (w584:bool)
          n333 = local read "5 5"() -> (w585:bool)
          n334 = local read "6 5"() -> (w586:bool)
          n335 = local read "7 5"() -> (w587:bool)
          n336 = local read "8 5"() -> (w588:bool)
          n337 = local read "9 5"() -> (w490:bool)
          n338 = local read "10 5"() -> (w489:bool)
          n339 = local read "9 6"() -> (w488:bool)
          n340 = local read "10 6"() -> (w487:bool)
          n341 = Build Array(w573, w574, w575, w576, w577, w578, w580, w579, w581, w582, w583, w584, w585, w586, w587, w588, w490, w489, w488, w487) -> (w521:bool[])
          n342 = local read "1 4"() -> (w557:bool)
          n343 = local read "2 4"() -> (w558:bool)
          n344 = local read "3 4"() -> (w559:bool)
          n345 = local read "4 4"() -> (w560:bool)
          n346 = local read "5 4"() -> (w561:bool)
          n347 = local read "6 4"() -> (w562:bool)
          n348 = local read "7 4"() -> (w563:bool)
          n349 = local read "8 4"() -> (w564:bool)
          n350 = local read "1 3"() -> (w565:bool)
          n351 = local read "2 3"() -> (w566:bool)
          n352 = local read "3 3"() -> (w567:bool)
          n353 = local read "4 3"() -> (w568:bool)
          n354 = local read "5 3"() -> (w569:bool)
          n355 = local read "6 3"() -> (w570:bool)
          n356 = local read "7 3"() -> (w571:bool)
          n357 = local read "8 3"() -> (w572:bool)
          n358 = local read "9 3"() -> (w494:bool)
          n359 = local read "10 3"() -> (w493:bool)
          n360 = local read "9 4"() -> (w492:bool)
          n361 = local read "10 4"() -> (w491:bool)
          n362 = Build Array(w557, w558, w559, w560, w561, w562, w563, w564, w565, w566, w567, w568, w569, w570, w571, w572, w494, w493, w492, w491) -> (w520:bool[])
          n363 = local read "1 2"() -> (w541:bool)
          n364 = local read "2 2"() -> (w542:bool)
          n365 = local read "3 2"() -> (w543:bool)
          n366 = local read "4 2"() -> (w544:bool)
          n367 = local read "5 2"() -> (w545:bool)
          n368 = local read "6 2"() -> (w546:bool)
          n369 = local read "7 2"() -> (w547:bool)
          n370 = local read "8 2"() -> (w548:bool)
          n371 = local read "1"() -> (w549:bool)
          n372 = local read "2"() -> (w550:bool)
          n373 = local read "3"() -> (w551:bool)
          n374 = local read "4"() -> (w552:bool)
          n375 = local read "5"() -> (w553:bool)
          n376 = local read "6"() -> (w554:bool)
          n377 = local read "7"() -> (w555:bool)
          n378 = local read "8"() -> (w556:bool)
          n379 = local read "9"() -> (w498:bool)
          n380 = local read "10"() -> (w497:bool)
          n381 = local read "9 2"() -> (w496:bool)
          n382 = local read "10 2"() -> (w495:bool)
          n383 = Build Array(w541, w542, w543, w544, w545, w546, w547, w548, w549, w550, w551, w552, w553, w554, w555, w556, w498, w497, w496, w495) -> (w531:bool[])
          n384 = local read "MCR  3"() -> (w480:bool)
          n385 = local read "MCL 3"() -> (w478:bool)
          n386 = local read "MCR 2"() -> (w464:bool)
          n387 = local read "MCL 2"() -> (w462:bool)
          n388 = local read "BCR 3"() -> (w475:bool)
          n389 = local read "TCR 3"() -> (w484:bool)
          n390 = local read "BCL 3"() -> (w473:bool)
          n391 = local read "MR  3"() -> (w486:bool)
          n392 = local read "TCL 3"() -> (w482:bool)
          n393 = local read "TCR 2"() -> (w458:bool)
          n394 = local read "BCR 2"() -> (w470:bool)
          n395 = local read "TCL 2"() -> (w457:bool)
          n396 = local read "MR  2"() -> (w466:bool)
          n397 = local read "BCL 2"() -> (w467:bool)
          n398 = local read "MC 3"() -> (w479:bool)
          n399 = local read "MC 2"() -> (w463:bool)
          n400 = local read "ML 3"() -> (w477:bool)
          n401 = local read "ML 2"() -> (w461:bool)
          n402 = local read "BC 3"() -> (w474:bool)
          n403 = local read "TC 3"() -> (w483:bool)
          n404 = local read "BR 3"() -> (w476:bool)
          n405 = local read "TR 3"() -> (w485:bool)
          n406 = local read "TC 2"() -> (w471:bool)
          n407 = local read "BC 2"() -> (w465:bool)
          n408 = local read "BL 3"() -> (w472:bool)
          n409 = local read "TL 3"() -> (w481:bool)
          n410 = local read "TR 2"() -> (w468:bool)
          n411 = local read "BR 2"() -> (w469:bool)
          n412 = local read "BL 2"() -> (w459:bool)
          n413 = local read "TL 2"() -> (w460:bool)
          n414 = Build Array(w471, w457, w458, w459, w460, w461, w462, w463, w464, w465, w466, w467, w468, w469, w470) -> (w456:bool[])
          n415 = Build Array(w472, w473, w474, w475, w476, w477, w478, w479, w480, w486, w481, w482, w483, w484, w485) -> (w450:bool[])
          n416 = local read "Player 1"() -> (w402:bool)
          n417 = local read "Player 2"() -> (w401:bool)
          n418 = local read "Player 3"() -> (w400:bool)
          n419 = local read "Player 4"() -> (w399:bool)
          n420 = local read "Pause"() -> (w524:bool)
          n421 = local read "W1"() -> (w532:bool)
          n422 = local read "W2"() -> (w533:bool)
          n423 = local read "1 7"() -> (w451:bool)
          n424 = local read "2 7"() -> (w538:bool)
          n425 = local read "3 7"() -> (w539:bool)
          n426 = local read "4 7"() -> (w540:bool)
          n427 = local read "5 7"() -> (w453:bool)
          n428 = local read "E1"() -> (w534:bool)
          n429 = local read "E2"() -> (w535:bool)
          n430 = local read "S1"() -> (w536:bool)
          n431 = local read "S2"() -> (w537:bool)
          n432 = local read "S3"() -> (w455:bool)
          n433 = local read "S4"() -> (w454:bool)
          n434 = Build Array(w402, w401, w532, w533, w534, w535, w536, w537, w451, w538, w539, w540, w524, w455, w454, w400, w399, w453) -> (w452:bool[])
          n435 = Build Array(w521, w520, w531, w456, w450, w452) -> (w529:bool[][])
          n436 = control-ref of="Player 1"() -> (w436:refnum<vi>)
          n437 = control-ref of="Player 2"() -> (w435:refnum<vi>)
          n438 = control-ref of="S3"() -> (w433:refnum<vi>)
          n439 = control-ref of="E1"() -> (w410:refnum<vi>)
          n440 = control-ref of="W1"() -> (w412:refnum<vi>)
          n441 = control-ref of="S2"() -> (w414:refnum<vi>)
          n442 = control-ref of="TL 3"() -> (w415:refnum<vi>)
          n443 = control-ref of="TC 3"() -> (w417:refnum<vi>)
          n444 = control-ref of="TR 3"() -> (w419:refnum<vi>)
          n445 = control-ref of="ML 3"() -> (w421:refnum<vi>)
          n446 = control-ref of="MC 3"() -> (w423:refnum<vi>)
          n447 = control-ref of="MR  3"() -> (w425:refnum<vi>)
          n448 = control-ref of="BL 3"() -> (w427:refnum<vi>)
          n449 = control-ref of="BC 3"() -> (w429:refnum<vi>)
          n450 = control-ref of="BR 3"() -> (w431:refnum<vi>)
          n451 = control-ref of="TCL 2"() -> (w438:refnum<vi>)
          n452 = control-ref of="TCR 2"() -> (w440:refnum<vi>)
          n453 = control-ref of="MCL 2"() -> (w442:refnum<vi>)
          n454 = control-ref of="MCR 2"() -> (w444:refnum<vi>)
          n455 = control-ref of="BCL 2"() -> (w446:refnum<vi>)
          n456 = control-ref of="BCR 2"() -> (w448:refnum<vi>)
          n457 = control-ref of="Name 1"() -> (w406:refnum<vi>)
          n458 = control-ref of="Name 2"() -> (w404:refnum<vi>)
          n459 = Or Array Elements(Boolean array=w529) -> (logical OR=w530:bool)
          n460 = control-ref of="Player 3"() -> (w437:refnum<vi>)
          n461 = control-ref of="Player 4"() -> (w434:refnum<vi>)
          n462 = control-ref of="S1"() -> (w407:refnum<vi>)
          n463 = control-ref of="E2"() -> (w411:refnum<vi>)
          n464 = control-ref of="W2"() -> (w413:refnum<vi>)
          n465 = control-ref of="S4"() -> (w408:refnum<vi>)
          n466 = control-ref of="TL 2"() -> (w416:refnum<vi>)
          n467 = control-ref of="TC 2"() -> (w418:refnum<vi>)
          n468 = control-ref of="TR 2"() -> (w420:refnum<vi>)
          n469 = control-ref of="ML 2"() -> (w422:refnum<vi>)
          n470 = control-ref of="MC 2"() -> (w424:refnum<vi>)
          n471 = control-ref of="MR  2"() -> (w426:refnum<vi>)
          n472 = control-ref of="BL 2"() -> (w428:refnum<vi>)
          n473 = control-ref of="BC 2"() -> (w430:refnum<vi>)
          n474 = control-ref of="BR 2"() -> (w432:refnum<vi>)
          n475 = control-ref of="TCL 3"() -> (w439:refnum<vi>)
          n476 = control-ref of="TCR 3"() -> (w441:refnum<vi>)
          n477 = control-ref of="MCL 3"() -> (w443:refnum<vi>)
          n478 = control-ref of="MCR  3"() -> (w445:refnum<vi>)
          n479 = control-ref of="BCL 3"() -> (w447:refnum<vi>)
          n480 = control-ref of="BCR 3"() -> (w449:refnum<vi>)
          n481 = control-ref of="Name 3"() -> (w405:refnum<vi>)
          n482 = control-ref of="Name 4"() -> (w403:refnum<vi>)
          n483 = local read "Video Frame"() -> (w522:u32)
          n484 = Build Array(w436, w437, w435, w434, w433, w407, w410, w411, w412, w413, w414, w408, w415, w416, w417, w418, w419, w420, w421, w422, w423, w424, w425, w426, w427, w428, w429, w430, w431, w432, w438, w439, w440, w441, w442, w443, w444, w445, w446, w447, w448, w449, w406, w405, w404, w403) -> (w409:refnum<vi>[])
          n485 = Array Size(array=w409) -> (size(s)=w526:i32)
          n486 = Divide(x=w526, y=2) -> (x/y=w528:dbl)
          n487 = case shown="True" w530 {
            tunnel: w522 -> [_ w633]
            tunnel: w590 -> [w606 w634]
            tunnel: [w606 w622] -> w511
            tunnel: w523 -> [_ w624]
            frame False {
            }
            frame True {
              n488 = stacked-sequence {
                tunnel: [_ _ w741 _ _ _ _ _ _] -> w639
                tunnel: [_ _ w740 _ _ _ _ _ _] -> w676
                tunnel: [_ _ w739 _ _ _ _ _ _] -> w675
                tunnel: [_ _ w738 _ _ _ _ _ _] -> w674
                tunnel: [_ _ w737 _ _ _ _ _ _] -> w673
                tunnel: [_ _ w736 _ _ _ _ _ _] -> w672
                tunnel: [_ _ w735 _ _ _ _ _ _] -> w671
                tunnel: [_ _ w734 _ _ _ _ _ _] -> w665
                tunnel: [_ _ w733 _ _ _ _ _ _] -> w670
                tunnel: [_ _ w732 _ _ _ _ _ _] -> w669
                tunnel: [_ _ w731 _ _ _ _ _ _] -> w668
                tunnel: [_ _ w730 _ _ _ _ _ _] -> w667
                tunnel: [_ _ w729 _ _ _ _ _ _] -> w666
                tunnel: [_ _ w728 _ _ _ _ _ _] -> w664
                tunnel: [_ _ w727 _ _ _ _ _ _] -> w663
                tunnel: [_ _ _ w789 _ _ _ _ _] -> w662
                tunnel: [_ _ _ w788 _ _ _ _ _] -> w661
                tunnel: [_ _ _ w787 _ _ _ _ _] -> w660
                tunnel: [_ _ _ _ w873 _ _ _ _] -> w659
                tunnel: [_ _ _ _ w872 _ _ _ _] -> w658
                tunnel: [_ _ _ _ w865 _ _ _ _] -> w657
                tunnel: [_ _ _ _ w864 _ _ _ _] -> w656
                tunnel: [_ _ _ _ w863 _ _ _ _] -> w655
                tunnel: [_ _ _ _ w862 _ _ _ _] -> w654
                tunnel: [_ _ _ _ w861 _ _ _ _] -> w653
                tunnel: [_ _ _ _ w860 _ _ _ _] -> w652
                tunnel: [_ _ _ _ w859 _ _ _ _] -> w651
                tunnel: [_ _ _ _ w858 _ _ _ _] -> w650
                tunnel: [_ _ _ _ w857 _ _ _ _] -> w649
                tunnel: [_ _ _ _ w856 _ _ _ _] -> w648
                tunnel: [_ _ _ _ _ _ _ w1001 _] -> w647
                tunnel: [_ _ _ _ _ _ _ w1000 _] -> w646
                tunnel: [_ _ _ _ _ _ _ w999 _] -> w645
                tunnel: [_ _ _ _ _ _ _ w998 _] -> w644
                tunnel: [_ _ _ _ _ _ _ w997 _] -> w643
                tunnel: [_ _ _ _ _ _ _ w996 _] -> w642
                tunnel: [_ _ _ _ _ _ w990 _ _] -> w641
                tunnel: [_ _ _ _ _ _ w990 _ _] -> w640
                tunnel: w634 -> [_ _ _ _ _ _ _ w1015 _]
                tunnel: [_ _ _ _ _ _ _ w1013 _] -> w629
                tunnel: w633 -> [w686 _ _ _ _ _ _ w1014 _]
                tunnel: [w686 _ _ _ _ _ _ _ _] -> w632
                tunnel: w624 -> [w685 _ _ _ _ _ _ _ _]
                tunnel: [w680 _ _ _ _ _ _ _ _] -> w623
                tunnel: [_ _ _ _ _ _ w989 _ _] -> w621
                tunnel: [_ _ _ _ _ _ w988 _ _] -> w620
                tunnel: [_ _ _ _ _ _ w987 _ _] -> w619
                tunnel: [_ _ _ _ _ _ w986 _ _] -> w618
                tunnel: [_ _ _ _ _ _ w985 _ _] -> w617
                tunnel: [_ _ _ _ _ _ w984 _ _] -> w616
                tunnel: [_ _ _ _ _ _ w983 _ _] -> w615
                tunnel: [_ _ _ _ _ _ w982 _ _] -> w614
                tunnel: [_ _ _ _ _ _ w981 _ _] -> w613
                tunnel: [_ _ _ _ _ w920 _ _ _] -> w612
                tunnel: [_ _ _ _ _ w922 _ _ _] -> w611
                tunnel: [_ _ _ _ _ _ w968 _ _] -> w610
                tunnel: [_ _ _ _ _ _ w967 _ _] -> w609
                tunnel: [_ _ _ _ _ _ w966 _ _] -> w608
                tunnel: [_ _ _ _ _ _ w965 _ _] -> w607
                frame #0 {
                  n489 = local read "Pause"() -> (w683:bool)
                  n490 = Tick Count (ms)() -> (millisecond timer value=w681:u32)
                  n491 = And(x=w683, y="Pause lag on") -> (x .and. y?=w684:bool)
                  n492 = case shown="True" w684 {
                    tunnel: w686 -> [_ w703]
                    tunnel: w685 -> [_ w705]
                    tunnel: ["pauselag" ("Image Name") w701] -> w680
                    frame False {
                    }
                    frame True {
                      w706 = T5 4 items=["Grayscale (U8)", "Grayscale (I16)", "Grayscale (SGL)", "Complex (CSG)", "RGB (U32)", "HSL (U32)", "RGB (U64)"] ("Image Type")
                      n493 = local read "framesPerSecond"() -> (w712:u32)
                      n494 = local read "Number of Frames"() -> (w702:u32)
                      n495 = Increment(x=w703) -> (x+1=w704:u32)
                      n496 = Multiply(x="Pause lag(s)", y=w712) -> (x*y=w710:dbl)
                      n497 = call "IMAQ Create"("Image Name"="pauselag", "Image Type"=w706) -> ("New Image"=w701:T1, "error out"=w707:errorcluster)  [unwired: 3 in]
                      n498 = Round Toward +Infinity(x=w710) -> (ceil(x): smallest int >= x=w709:dbl)
                      n499 = for {
                        N: w709 -> [_]
                        tunnel: w704 -> [w719]
                        tunnel: w707 -> [w722]
                        tunnel: w701 -> [w721]
                        tunnel: w705 -> [w718]
                        tunnel: w702 -> [w716]
                        i -> [w720]
                        n500 = Add(x=w720, y=w719) -> (x+y=w715:u32)
                        n501 = local read "playback speed"() -> (w713:dbl)
                        n502 = Less Or Equal?(x=w716, y=w715) -> (x <= y?=w717:bool)
                        n503 = Select(t=w716, s=w717, f=w715) -> (s? t:f=w714:u32)
                        n504 = call "IMAQ AVI Read Frame"("error in (no error)"=w722, "Frame Number"=w714, "Image"=w721, "Avi Refnum"=w718) -> ("Image Out"=w723:T1)  [unwired: 4 in, 3 out]
                        n505 = local write "Video"(w723) -> ()
                        n506 = Wait (ms)(milliseconds to wait=w713) -> ()  [unwired: 1 out]
                      }
                    }
                  }
                  n507 = while {
                    tunnel: w681 -> [w698]
                    i -> [w689]
                    stop <- w696 stop-if-true
                    w692 = u32 25 ("milliseconds to wait")
                    n508 = Tick Count (ms)() -> (millisecond timer value=w699:u32)
                    n509 = Subtract(x=w699, y=w698) -> (x-y=w697:u32)
                    n510 = Multiply(x="Code lag(s)", y=1000) -> (x*y=w693:dbl)
                    n511 = Greater Or Equal?(x=w697, y=w693) -> (x >= y?=w696:bool)
                    n512 = Divide(x=w693, y=w692) -> (x/y=w691:dbl)
                    n513 = Divide(x=300.0, y=w691) -> (x/y=w688:dbl)
                    n514 = Multiply(x=w689, y=w688) -> (x*y=→"task":dbl)
                    n515 = Wait (ms)(milliseconds to wait=w692) -> ()  [unwired: 1 out]
                  }
                }
                frame #1 {
                  n516 = while {
                    stop <- w724 continue-if-true
                    n517 = local read "START"() -> (w725:bool)
                    n518 = local read "Pause"() -> (w726:bool)
                    n519 = And(x=w725, y=w726) -> (x .and. y?=w724:bool)
                  }
                }
                frame #2 {
                  n520 = Or(x="BC 3", y="BC 2") -> (x .or. y?=w761:bool)
                  n521 = Or(x="BL 3", y="BL 2") -> (x .or. y?=w762:bool)
                  n522 = Or(x="BR 2", y="BR 3") -> (x .or. y?=w760:bool)
                  n523 = Or(x="TC 2", y="TC 3") -> (x .or. y?=w767:bool)
                  n524 = Or(x="TL 3", y="TL 2") -> (x .or. y?=w768:bool)
                  n525 = Or(x="TR 2", y="TR 3") -> (x .or. y?=w766:bool)
                  n526 = Boolean To (0,1)(Boolean=w762) -> (0, 1=w731:i16)
                  n527 = Boolean To (0,1)(Boolean=w760) -> (0, 1=w727:i16)
                  n528 = Boolean To (0,1)(Boolean=w768) -> (0, 1=w741:i16)
                  n529 = Boolean To (0,1)(Boolean=w761) -> (0, 1=w729:i16)
                  n530 = Boolean To (0,1)(Boolean=w766) -> (0, 1=w737:i16)
                  n531 = Boolean To (0,1)(Boolean=w767) -> (0, 1=w739:i16)
                  n532 = Or(x="TCL 2", y="TCL 3") -> (x .or. y?=w759:bool)
                  n533 = Or(x="BCL 2", y="BCL 3") -> (x .or. y?=w748:bool)
                  n534 = Or(x="BCR 2", y="BCR 3") -> (x .or. y?=w749:bool)
                  n535 = Or(x="TCR 2", y="TCR 3") -> (x .or. y?=w756:bool)
                  n536 = Boolean To (0,1)(Boolean=w759) -> (0, 1=w740:i16)
                  n537 = Or(x="ML 3", y="ML 2") -> (x .or. y?=w765:bool)
                  n538 = Boolean To (0,1)(Boolean=w748) -> (0, 1=w730:i16)
                  n539 = Boolean To (0,1)(Boolean=w749) -> (0, 1=w728:i16)
                  n540 = Or(x="MR  2", y="MR  3") -> (x .or. y?=w763:bool)
                  n541 = Boolean To (0,1)(Boolean=w756) -> (0, 1=w738:i16)
                  n542 = Or(x="MC 2", y="MC 3") -> (x .or. y?=w764:bool)
                  n543 = Boolean To (0,1)(Boolean=w765) -> (0, 1=w736:i16)
                  n544 = Boolean To (0,1)(Boolean=w764) -> (0, 1=w734:i16)
                  n545 = Boolean To (0,1)(Boolean=w763) -> (0, 1=w732:i16)
                  n546 = Or(x="MCL 2", y="MCL 3") -> (x .or. y?=w754:bool)
                  n547 = Or(x="MCR 2", y="MCR  3") -> (x .or. y?=w752:bool)
                  n548 = Boolean To (0,1)(Boolean=w754) -> (0, 1=w735:i16)
                  n549 = Boolean To (0,1)(Boolean=w752) -> (0, 1=w733:i16)
                }
                frame #3 {
                  n550 = Build Array("1", "2", "3", "4", "5", "6", "7", "8", "9", "10", "1 2", "2 2", "3 2", "4 2", "5 2", "6 2", "7 2", "8 2", "9 2", "10 2") -> (w847:bool[])
                  "FH" <- w847
                  n551 = Or Array Elements(Boolean array=w847) -> (logical OR=w845:bool)
                  n552 = Boolean To (0,1)(Boolean=w845) -> (0, 1=w789:i16)
                  n553 = Build Array("1 3", "2 3", "3 3", "4 3", "5 3", "6 3", "7 3", "8 3", "9 3", "10 3", "1 4", "2 4", "3 4", "4 4", "5 4", "6 4", "7 4", "8 4", "9 4", "10 4") -> (w846:bool[])
                  "BH" <- w846
                  n554 = Or Array Elements(Boolean array=w846) -> (logical OR=w844:bool)
                  n555 = Boolean To (0,1)(Boolean=w844) -> (0, 1=w788:i16)
                  n556 = Build Array("1 5", "2 5", "3 5", "4 5", "5 5", "6 5", "7 5", "8 5", "9 5", "10 5", "1 6", "2 6", "3 6", "4 6", "5 6", "6 6", "7 6", "8 6", "9 6", "10 6") -> (w810:bool[])
                  "OH" <- w810
                  n557 = Or Array Elements(Boolean array=w810) -> (logical OR=w843:bool)
                  n558 = Boolean To (0,1)(Boolean=w843) -> (0, 1=w787:i16)
                }
                frame #4 {
                  w912 = 10 ("index")
                  n559 = local read "OH"() -> (w903:bool[])
                  n560 = local read "BH"() -> (w904:bool[])
                  n561 = local read "FH"() -> (w905:bool[])
                  n562 = Split 1D Array(array=w905, index=w912) -> (first subarray=w901:bool[], second subarray=w902:bool[])
                  n563 = Split 1D Array(array=w904, index=w912) -> (first subarray=w911:bool[], second subarray=w909:bool[])
                  n564 = Split 1D Array(array=w903, index=w912) -> (first subarray=w910:bool[], second subarray=w908:bool[])
                  n565 = Build Array(w901, w911, w910) -> (w900:bool[][])
                  n566 = Build Array(w902, w909, w908) -> (w899:bool[][])
                  n567 = Or Array Elements(Boolean array=w900) -> (logical OR=w907:bool)
                  n568 = Or Array Elements(Boolean array=w899) -> (logical OR=w906:bool)
                  n569 = Insert Into Array(array=w900, new element=w899) -> (w898:bool[][])  [unwired: 2 in]
                  n570 = Boolean To (0,1)(Boolean=w907) -> (0, 1=w873:i16)
                  n571 = Boolean To (0,1)(Boolean=w906) -> (0, 1=w872:i16)
                  n572 = Index Array(array=w898, index (col) #1=3 ("disabled index (col)"), index (col) #2=2 ("index (col)"), index (col) #3=5 ("index (col)"), index (col) #4=0 ("index (col)"), index (col) #5=7 ("index (col)"), index (col) #6=4 ("index (col)"), index (col) #7=8 ("index (col)"), index (col) #8=9 ("index (col)"), index (col) #9=1 ("index (col)"), index (col) #10=6 ("index (col)")) -> (element #1=w888:bool[], element #2=w880:bool[], element #3=w879:bool[], element #4=w878:bool[], element #5=w877:bool[], element #6=w876:bool[], element #7=w875:bool[], element #8=w874:bool[], element #9=w867:bool[], element #10=w866:bool[])  [unwired: 10 in]
                  n573 = Or Array Elements(Boolean array=w888) -> (logical OR=w889:bool)
                  n574 = Or Array Elements(Boolean array=w879) -> (logical OR=w885:bool)
                  n575 = Or Array Elements(Boolean array=w877) -> (logical OR=w884:bool)
                  n576 = Or Array Elements(Boolean array=w875) -> (logical OR=w881:bool)
                  n577 = Or Array Elements(Boolean array=w867) -> (logical OR=w869:bool)
                  n578 = Or Array Elements(Boolean array=w880) -> (logical OR=w887:bool)
                  n579 = Or Array Elements(Boolean array=w878) -> (logical OR=w886:bool)
                  n580 = Or Array Elements(Boolean array=w876) -> (logical OR=w883:bool)
                  n581 = Or Array Elements(Boolean array=w874) -> (logical OR=w882:bool)
                  n582 = Or Array Elements(Boolean array=w866) -> (logical OR=w868:bool)
                  n583 = Boolean To (0,1)(Boolean=w889) -> (0, 1=w865:i16)
                  n584 = Boolean To (0,1)(Boolean=w885) -> (0, 1=w863:i16)
                  n585 = Boolean To (0,1)(Boolean=w884) -> (0, 1=w861:i16)
                  n586 = Boolean To (0,1)(Boolean=w881) -> (0, 1=w859:i16)
                  n587 = Boolean To (0,1)(Boolean=w869) -> (0, 1=w857:i16)
                  n588 = Boolean To (0,1)(Boolean=w887) -> (0, 1=w864:i16)
                  n589 = Boolean To (0,1)(Boolean=w886) -> (0, 1=w862:i16)
                  n590 = Boolean To (0,1)(Boolean=w883) -> (0, 1=w860:i16)
                  n591 = Boolean To (0,1)(Boolean=w882) -> (0, 1=w858:i16)
                  n592 = Boolean To (0,1)(Boolean=w868) -> (0, 1=w856:i16)
                }
                frame #5 {
                  w919 = i16 1 ("t")
                  n593 = local read "MCR  3"() -> (w951:bool)
                  n594 = local read "MCL 3"() -> (w943:bool)
                  n595 = local read "BCR 3"() -> (w955:bool)
                  n596 = local read "TCR 3"() -> (w946:bool)
                  n597 = local read "BCL 3"() -> (w957:bool)
                  n598 = local read "MR  3"() -> (w950:bool)
                  n599 = local read "TCL 3"() -> (w948:bool)
                  n600 = local read "MC 3"() -> (w952:bool)
                  n601 = local read "ML 3"() -> (w953:bool)
                  n602 = local read "BC 3"() -> (w956:bool)
                  n603 = local read "TC 3"() -> (w947:bool)
                  n604 = local read "BR 3"() -> (w954:bool)
                  n605 = local read "TR 3"() -> (w945:bool)
                  n606 = local read "BL 3"() -> (w958:bool)
                  n607 = local read "TL 3"() -> (w949:bool)
                  n608 = local read "S1"() -> (w918:bool)
                  n609 = local read "S2"() -> (w917:bool)
                  n610 = local read "S3"() -> (w916:bool)
                  n611 = local read "S4"() -> (w915:bool)
                  n612 = Or(x=w916, y=w915) -> (x .or. y?=w913:bool)
                  n613 = Or(x=w918, y=w917) -> (x .or. y?=w914:bool)
                  n614 = Compound Arithmetic op=OR(w958, w957, w956, w955, w954, w953, w943, w952, w951, w950, w949, w948, w947, w946, w945) -> (w944:bool)
                  "P1 position" <- w944
                  n615 = local read "MCR 2"() -> (w936:bool)
                  n616 = local read "MCL 2"() -> (w933:bool)
                  n617 = local read "TCR 2"() -> (w929:bool)
                  n618 = local read "BCR 2"() -> (w942:bool)
                  n619 = local read "TCL 2"() -> (w927:bool)
                  n620 = local read "MR  2"() -> (w938:bool)
                  n621 = local read "BCL 2"() -> (w939:bool)
                  n622 = local read "MC 2"() -> (w935:bool)
                  n623 = local read "ML 2"() -> (w932:bool)
                  n624 = local read "TC 2"() -> (w934:bool)
                  n625 = local read "BC 2"() -> (w937:bool)
                  n626 = local read "TR 2"() -> (w940:bool)
                  n627 = local read "BR 2"() -> (w941:bool)
                  n628 = local read "BL 2"() -> (w930:bool)
                  n629 = local read "TL 2"() -> (w931:bool)
                  n630 = Compound Arithmetic op=OR(w927, w929, w930, w931, w932, w933, w934, w935, w936, w937, w938, w939, w940, w941, w942) -> (w928:bool)
                  "P2 position" <- w928
                  n631 = Compound Arithmetic op=OR(w944, "Player 1", "Player 2", w914) -> (w964:bool)
                  n632 = Compound Arithmetic op=OR(w928, "Player 3", "Player 4", w913) -> (w962:bool)
                  n633 = Boolean To (0,1)(Boolean=w962) -> (0, 1=w923:i16)
                  n634 = Boolean To (0,1)(Boolean=w964) -> (0, 1=w921:i16)
                  n635 = Equal To 0?(x=w923) -> (x = 0?=w925:bool)
                  n636 = Equal To 0?(x=w921) -> (x = 0?=w926:bool)
                  n637 = And(x=w926, y=w925) -> (x .and. y?=w924:bool)
                  n638 = Select(t=w919, s=w924, f=w921) -> (s? t:f=w920:i16)
                  n639 = Select(t=w919, s=w924, f=w923) -> (s? t:f=w922:i16)
                }
                frame #6 {
                  w990 = i16 0
                  n640 = local read "Player 1"() -> (w972:bool)
                  n641 = local read "Player 2"() -> (w971:bool)
                  n642 = local read "Player 3"() -> (w970:bool)
                  n643 = local read "Player 4"() -> (w969:bool)
                  n644 = Or(x="S1", y=w972) -> (x .or. y?=w979:bool)
                  n645 = Or(x="S2", y=w971) -> (x .or. y?=w980:bool)
                  n646 = Or(x="S3", y=w970) -> (x .or. y?=w977:bool)
                  n647 = Or(x="S4", y=w969) -> (x .or. y?=w978:bool)
                  n648 = Boolean To (0,1)(Boolean="S1") -> (0, 1=w989:i16)
                  n649 = Boolean To (0,1)(Boolean="S2") -> (0, 1=w988:i16)
                  n650 = Boolean To (0,1)(Boolean="S3") -> (0, 1=w987:i16)
                  n651 = Boolean To (0,1)(Boolean="S4") -> (0, 1=w986:i16)
                  n652 = Boolean To (0,1)(Boolean="1 7") -> (0, 1=w985:i16)
                  n653 = Boolean To (0,1)(Boolean="2 7") -> (0, 1=w984:i16)
                  n654 = Boolean To (0,1)(Boolean="3 7") -> (0, 1=w983:i16)
                  n655 = Boolean To (0,1)(Boolean="4 7") -> (0, 1=w982:i16)
                  n656 = Boolean To (0,1)(Boolean="5 7") -> (0, 1=w981:i16)
                  n657 = Boolean To (0,1)(Boolean=w979) -> (0, 1=w968:i16)
                  n658 = Boolean To (0,1)(Boolean=w980) -> (0, 1=w967:i16)
                  n659 = Boolean To (0,1)(Boolean=w977) -> (0, 1=w966:i16)
                  n660 = Boolean To (0,1)(Boolean=w978) -> (0, 1=w965:i16)
                }
                frame #7 {
                  n661 = local read "P1 position"() -> (w1022:bool)
                  n662 = local read "P2 position"() -> (w1018:bool)
                  n663 = local read "OH"() -> (w1023:bool[])
                  n664 = local read "BH"() -> (w1024:bool[])
                  n665 = local read "FH"() -> (w1025:bool[])
                  n666 = local read "Player 1"() -> (w1026:bool)
                  n667 = local read "Player 2"() -> (w1027:bool)
                  n668 = local read "Player 3"() -> (w1012:bool)
                  n669 = local read "Player 4"() -> (w1011:bool)
                  n670 = local read "1 7"() -> (w1006:bool)
                  n671 = local read "2 7"() -> (w1005:bool)
                  n672 = local read "3 7"() -> (w1004:bool)
                  n673 = local read "4 7"() -> (w1003:bool)
                  n674 = local read "5 7"() -> (w1002:bool)
                  n675 = local read "S1"() -> (w1010:bool)
                  n676 = local read "S2"() -> (w1009:bool)
                  n677 = local read "S3"() -> (w1008:bool)
                  n678 = local read "S4"() -> (w1007:bool)
                  n679 = Or Array Elements(Boolean array=w1025) -> (logical OR=w1021:bool)
                  n680 = Or Array Elements(Boolean array=w1024) -> (logical OR=w1020:bool)
                  n681 = Or Array Elements(Boolean array=w1023) -> (logical OR=w1019:bool)
                  n682 = Not(x="Link Errors") -> (.not. x?=w1028:bool)
                  n683 = Compound Arithmetic op=OR(w1028, w1022, w1021, w1020, w1019, w1018, w1026, w1027, w1012, w1011, w1010, w1009, w1008, w1007, w1006, w1005, w1004, w1003, w1002) -> (w1016:bool)
                  n684 = case shown="False" w1016 {
                    tunnel: [w1029 w1069] -> w1001
                    tunnel: [w1029 w1068] -> w1000
                    tunnel: [w1029 w1067] -> w999
                    tunnel: [w1029 w1066] -> w998
                    tunnel: [w1029 w1065] -> w997
                    tunnel: [w1029 w1064] -> w996
                    tunnel: w1015 -> [w1033 w1063]
                    tunnel: w1014 -> [w1052 _]
                    tunnel: [w1032 w1063] -> w1013
                    frame False {
                      w1029 = i16 0
                      n685 = local read "W1"() -> (w1048:bool)
                      n686 = local read "W2"() -> (w1049:bool)
                      n687 = local read "E1"() -> (w1050:bool)
                      n688 = local read "E2"() -> (w1051:bool)
                      n689 = Index Array(array=w1033, index (col)=0 ("disabled index (col)")) -> (element=w1053:i64[])  [unwired: 1 in]
                      n690 = for {
                        tunnel: w1053 -> [w1056] mode=indexing
                        tunnel: w1052 -> [w1057]
                        tunnel: [w1056] -> w1055 mode=indexing if=w1058
                        stop <- w1058 continue-if-true
                        n691 = Less Or Equal?(x=w1056, y=w1057) -> (x <= y?=w1058:bool)
                      }
                      n692 = Or(x=w1048, y=w1051) -> (x .or. y?=w1047:bool)
                      n693 = Or(x=w1049, y=w1050) -> (x .or. y?=w1046:bool)
                      n694 = Boolean To (0,1)(Boolean=w1048) -> (0, 1=w1043:i16)
                      n695 = Boolean To (0,1)(Boolean=w1049) -> (0, 1=w1042:i16)
                      n696 = Boolean To (0,1)(Boolean=w1050) -> (0, 1=w1037:i16)
                      n697 = Boolean To (0,1)(Boolean=w1051) -> (0, 1=w1036:i16)
                      n698 = Boolean To (0,1)(Boolean=w1047) -> (0, 1=w1035:i16)
                      n699 = Boolean To (0,1)(Boolean=w1046) -> (0, 1=w1034:i16)
                      n700 = Array Size(array=w1055) -> (size(s)=w1031:i32)
                      n701 = Decrement(x=w1031) -> (x-1=w1030:i32)
                      n702 = Replace Array Subset(array=w1033, new element #1=w1043, index (row) #1=w1030, index (col) #1=31 ("disabled index (col)"), new element #2=w1042, index (row) #2=w1030, index (col) #2=32 ("disabled index (col)"), new element #3=w1037, index (row) #3=w1030, index (col) #3=33 ("disabled index (col)"), new element #4=w1036, index (row) #4=w1030, index (col) #4=34 ("disabled index (col)"), new element #5=w1035, index (row) #5=w1030, index (col) #5=35 ("disabled index (col)"), new element #6=w1034, index (row) #6=w1030, index (col) #6=36 ("disabled index (col)")) -> (w1032:i64[][])
                    }
                    frame True {
                      n703 = Or(x="W1", y="E2") -> (x .or. y?=w1070:bool)
                      n704 = Or(x="E1", y="W2") -> (x .or. y?=w1071:bool)
                      n705 = Boolean To (0,1)(Boolean="W1") -> (0, 1=w1069:i16)
                      n706 = Boolean To (0,1)(Boolean="E1") -> (0, 1=w1068:i16)
                      n707 = Boolean To (0,1)(Boolean="W2") -> (0, 1=w1067:i16)
                      n708 = Boolean To (0,1)(Boolean="E2") -> (0, 1=w1066:i16)
                      n709 = Boolean To (0,1)(Boolean=w1070) -> (0, 1=w1065:i16)
                      n710 = Boolean To (0,1)(Boolean=w1071) -> (0, 1=w1064:i16)
                    }
                  }
                }
                frame #8 {
                  w1072 = FALSE ("4 6")
                  n711 = local write "1 6"(w1072) -> ()
                  n712 = local write "2 6"(w1072) -> ()
                  n713 = local write "3 6"(w1072) -> ()
                  n714 = local write "4 6"(w1072) -> ()
                  n715 = local write "5 6"(w1072) -> ()
                  n716 = local write "6 6"(w1072) -> ()
                  n717 = local write "7 6"(w1072) -> ()
                  n718 = local write "8 6"(w1072) -> ()
                  n719 = local write "9 6"(w1072) -> ()
                  n720 = local write "10 6"(w1072) -> ()
                  n721 = local write "Player 1"(w1072) -> ()
                  n722 = local write "Player 2"(w1072) -> ()
                  n723 = local write "Player 3"(w1072) -> ()
                  n724 = local write "Player 4"(w1072) -> ()
                  n725 = local write "1 5"(w1072) -> ()
                  n726 = local write "2 5"(w1072) -> ()
                  n727 = local write "3 5"(w1072) -> ()
                  n728 = local write "4 5"(w1072) -> ()
                  n729 = local write "5 5"(w1072) -> ()
                  n730 = local write "6 5"(w1072) -> ()
                  n731 = local write "7 5"(w1072) -> ()
                  n732 = local write "8 5"(w1072) -> ()
                  n733 = local write "9 5"(w1072) -> ()
                  n734 = local write "10 5"(w1072) -> ()
                  n735 = local write "W1"(w1072) -> ()
                  n736 = local write "W2"(w1072) -> ()
                  n737 = local write "E1"(w1072) -> ()
                  n738 = local write "E2"(w1072) -> ()
                  n739 = local write "1 4"(w1072) -> ()
                  n740 = local write "2 4"(w1072) -> ()
                  n741 = local write "3 4"(w1072) -> ()
                  n742 = local write "4 4"(w1072) -> ()
                  n743 = local write "5 4"(w1072) -> ()
                  n744 = local write "6 4"(w1072) -> ()
                  n745 = local write "7 4"(w1072) -> ()
                  n746 = local write "8 4"(w1072) -> ()
                  n747 = local write "9 4"(w1072) -> ()
                  n748 = local write "10 4"(w1072) -> ()
                  n749 = local write "1 3"(w1072) -> ()
                  n750 = local write "2 3"(w1072) -> ()
                  n751 = local write "3 3"(w1072) -> ()
                  n752 = local write "4 3"(w1072) -> ()
                  n753 = local write "5 3"(w1072) -> ()
                  n754 = local write "6 3"(w1072) -> ()
                  n755 = local write "7 3"(w1072) -> ()
                  n756 = local write "8 3"(w1072) -> ()
                  n757 = local write "9 3"(w1072) -> ()
                  n758 = local write "10 3"(w1072) -> ()
                  n759 = local write "S1"(w1072) -> ()
                  n760 = local write "S2"(w1072) -> ()
                  n761 = local write "S3"(w1072) -> ()
                  n762 = local write "S4"(w1072) -> ()
                  n763 = local write "1 7"(w1072) -> ()
                  n764 = local write "2 7"(w1072) -> ()
                  n765 = local write "3 7"(w1072) -> ()
                  n766 = local write "4 7"(w1072) -> ()
                  n767 = local write "5 7"(w1072) -> ()
                  n768 = local write "1 2"(w1072) -> ()
                  n769 = local write "2 2"(w1072) -> ()
                  n770 = local write "3 2"(w1072) -> ()
                  n771 = local write "4 2"(w1072) -> ()
                  n772 = local write "5 2"(w1072) -> ()
                  n773 = local write "6 2"(w1072) -> ()
                  n774 = local write "7 2"(w1072) -> ()
                  n775 = local write "8 2"(w1072) -> ()
                  n776 = local write "9 2"(w1072) -> ()
                  n777 = local write "10 2"(w1072) -> ()
                  n778 = local write "1"(w1072) -> ()
                  n779 = local write "2"(w1072) -> ()
                  n780 = local write "3"(w1072) -> ()
                  n781 = local write "4"(w1072) -> ()
                  n782 = local write "5"(w1072) -> ()
                  n783 = local write "6"(w1072) -> ()
                  n784 = local write "7"(w1072) -> ()
                  n785 = local write "8"(w1072) -> ()
                  n786 = local write "9"(w1072) -> ()
                  n787 = local write "10"(w1072) -> ()
                  n788 = local write "TC 2"(w1072) -> ()
                  n789 = local write "TCL 2"(w1072) -> ()
                  n790 = local write "TCR 2"(w1072) -> ()
                  n791 = local write "BL 2"(w1072) -> ()
                  n792 = local write "TL 2"(w1072) -> ()
                  n793 = local write "ML 2"(w1072) -> ()
                  n794 = local write "MCL 2"(w1072) -> ()
                  n795 = local write "MC 2"(w1072) -> ()
                  n796 = local write "MCR 2"(w1072) -> ()
                  n797 = local write "BC 2"(w1072) -> ()
                  n798 = local write "MR  2"(w1072) -> ()
                  n799 = local write "BCL 2"(w1072) -> ()
                  n800 = local write "TR 2"(w1072) -> ()
                  n801 = local write "BR 2"(w1072) -> ()
                  n802 = local write "BCR 2"(w1072) -> ()
                  n803 = local write "BL 3"(w1072) -> ()
                  n804 = local write "BCL 3"(w1072) -> ()
                  n805 = local write "BC 3"(w1072) -> ()
                  n806 = local write "BCR 3"(w1072) -> ()
                  n807 = local write "BR 3"(w1072) -> ()
                  n808 = local write "ML 3"(w1072) -> ()
                  n809 = local write "MCL 3"(w1072) -> ()
                  n810 = local write "MC 3"(w1072) -> ()
                  n811 = local write "MCR  3"(w1072) -> ()
                  n812 = local write "MR  3"(w1072) -> ()
                  n813 = local write "TL 3"(w1072) -> ()
                  n814 = local write "TCL 3"(w1072) -> ()
                  n815 = local write "TC 3"(w1072) -> ()
                  n816 = local write "TCR 3"(w1072) -> ()
                  n817 = local write "TR 3"(w1072) -> ()
                }
              }
              n818 = Build Array(w632, w639, w676, w675, w674, w673, w672, w671, w665, w670, w669, w668, w667, w666, w664, w663, w662, w661, w660, w659, w658, w657, w656, w655, w654, w653, w652, w651, w650, w649, w648, w647, w646, w645, w644, w643, w642, w641, w640, w621, w620, w619, w618, w617, w616, w615, w614, w613, w612, w611, w610, w609, w608, w607) -> (w628:u32[])
              n819 = call "IMAQ Dispose"("Image"=w623) -> ()  [unwired: 5 in, 1 out]
              n820 = Index Array(array=w629, index (col)=0 ("disabled index (col)")) -> (element=w638:i64[])  [unwired: 1 in]
              n821 = Delete From Array(array=w628, index=0) -> (array with subset deleted=w630:u32[])  [unwired: 1 in, 1 out]
              n822 = for {
                tunnel: w638 -> [w677] mode=indexing
                tunnel: w632 -> [w678]
                tunnel: [w677] -> w636 mode=indexing if=w679
                stop <- w679 continue-if-true
                n823 = Less Or Equal?(x=w677, y=w678) -> (x <= y?=w679:bool)
              }
              n824 = Array Max & Min(array=w630) -> (max value=w627:u32)  [unwired: 3 out]
              n825 = Equal To 0?(x=w627) -> (x = 0?=w625:bool)
              n826 = Array Size(array=w636) -> (size(s)=w635:i32)
              n827 = Insert Into Array(array=w629, index (row)=w635, new element=w628) -> (w626:i64[][])  [unwired: 1 in]
              n828 = Select(t=w629, s=w625, f=w626) -> (s? t:f=w622:i64[][])
            }
          }
          n829 = case shown="True" "Switch position" {
            tunnel: w409 -> [_ w593]
            tunnel: w528 -> [_ w592]
            frame False {
            }
            frame True {
              n830 = for {
                N: w592 -> [_]
                tunnel: w593 -> [w600]
                i -> [w599]
                n831 = Multiply(x=2, y=w599) -> (x*y=w597:i32)
                n832 = Increment(x=w597) -> (x+1=w596:i32)
                n833 = Index Array(array=w600, index #1=w597, index #2=w596) -> (element #1=w594:refnum<vi>, element #2=w595:refnum<vi>)
                n834 = property class="Ctl"(reference=w594) -> (error out=w605:errorcluster, "Position"=w602:T8)  [unwired: 1 in, 1 out]
                n835 = property class="Ctl"(reference=w595, error in=w605) -> (error out=w604:errorcluster, "Position"=w601:T8)  [unwired: 1 out]
                n836 = property class="Ctl"(reference=w595, error in=w604, "Position"=w602) -> (error out=w603:errorcluster)  [unwired: 1 out]
                n837 = property class="Ctl"(reference=w594, error in=w603, "Position"=w601) -> ()  [unwired: 2 out]
              }
              n838 = local write "Switch position"(FALSE ("Switch position")) -> ()
            }
          }
          n839 = Build Array("Name 1", "Name 2", "Name 3", "Name 4") -> (w499:string[])
          n840 = call "EVENTS(SubVI).vi"() -> ("Events"=w505:string)  [unwired: 1 in]
          n841 = local read "Video file"() -> (w514:path)
          n842 = local read "Data file"() -> (w507:path)
          n843 = call "Doubles Events (SubVI).vi"("Singles Events"=w505, "PLAYER NAMES"=w499) -> ("Edited Events For Doubles"=w504:string)
          n844 = call <vilib>:"Get File Extension.vi"("file"=w514) -> ("filename without extension"=w516:string)  [unwired: 7 in, 3 out]
          n845 = Array To Spreadsheet String(delimiter (Tab)="\t" ("delimiter (\\t)"), array=w511, 3:"%.3f" ("format (%.3f)")) -> (spreadsheet string=w519:string)
          n846 = Open/Create/Replace File(file path (use dialog)=w507, operation (0:open)=T3."replace") -> (refnum out=w509:refnum<file>, error out=w508:errorcluster)  [unwired: 4 in, 1 out]
          n847 = Concatenate Strings("avi file" ("string"), w517, w516, w517, w517, w504, w519) -> (w518:string)
          n848 = Write to Text File(file (use dialog)=w509, text=w518, error in=w508) -> (refnum out=w506:refnum<file>)  [unwired: 1 in, 2 out]
          "coding" <- w590
        }
        frame "Display" {
          n849 = stacked-sequence {
            tunnel: w1079 -> [w1175 w1414]
            frame #0 {
              w1165 = i64 0 ("new element/subarray")
              w1164 = i64 0 ("new element/subarray")
              w1163 = i64 0 ("new element/subarray")
              w1135 = 0.0 ("disabled index (col)")
              n850 = Index Array(array=w1175, index (col) #1=39 ("length"), index (col) #2=40 ("disabled index (col)"), index (col) #3=41 ("index (col)"), index (col) #4=42 ("index (col)"), index (col) #5=35 ("index (col)"), index (col) #6=36 ("index (col)")) -> (element #1=w1155:i64[], element #2=w1156:i64[], element #3=w1084:i64[], element #4=w1083:i64[], element #5=w1088:i64[], element #6=w1087:i64[])  [unwired: 6 in]
              n851 = Index Array(array=w1175, index (col)=0 ("disabled index (col)")) -> (element=w1100:i64[])  [unwired: 1 in]
              n852 = Or(x=w1088, y=w1087) -> (x .or. y?=w1112:i64[])
              n853 = Compound Arithmetic op=OR(w1155, w1156, w1084, w1083) -> (w1157:i64[])
              n854 = for {
                shift-right: [w1209] -> _
                shift-left: w1135 -> [w1208]
                shift-right: [w1207] -> _
                shift-left: w1135 -> [w1206]
                tunnel: w1087 -> [w1212] mode=indexing
                tunnel: w1088 -> [w1219] mode=indexing
                tunnel: [w1203] -> w1098 mode=indexing if=w1201
                tunnel: [w1202] -> w1099 mode=indexing if=w1201
                w1211 = 1.0 ("x")
                w1216 = 1.0 ("x")
                n855 = Equal?(x=w1216, y=w1219) -> (x = y?=w1213:bool)
                n856 = Add(x=w1206, y=w1211) -> (x+y=w1210:dbl)
                n857 = Add(x=w1216, y=w1208) -> (x+y=w1215:dbl)
                n858 = Equal?(x=w1212, y=w1211) -> (x = y?=w1218:bool)
                n859 = Or(x=w1213, y=w1218) -> (x .or. y?=w1201:bool)
                n860 = Select(t=0.0, s=w1218, f=w1215) -> (s? t:f=w1204:dbl)
                n861 = Select(t=0.0, s=w1213, f=w1210) -> (s? t:f=w1202:dbl)
                n862 = Multiply(x=-1.0 ("y"), y=w1204) -> (x*y=w1203:dbl)
                n863 = Select(t=w1204, s=w1201, f=w1208) -> (s? t:f=w1209:dbl)
                n864 = Select(t=w1202, s=w1201, f=w1206) -> (s? t:f=w1207:dbl)
              }
              "p1y" <- w1098
              "p2y" <- w1099
              n865 = for {
                tunnel: w1157 -> [w1292] mode=indexing
                tunnel: w1100 -> [w1289] mode=indexing
                tunnel: [w1289] -> w1113 mode=indexing if=w1291
                tunnel: w1112 -> [w1290] mode=indexing
                tunnel: [w1289] -> w1111 mode=indexing if=w1288
                w1287 = 1.0 ("x")
                n866 = Equal?(x=w1287, y=w1292) -> (x = y?=w1291:bool)
                n867 = Equal?(x=w1287, y=w1290) -> (x = y?=w1288:bool)
              }
              "service frames" <- w1113
              "point frames" <- w1111
              n868 = for {
                tunnel: w1088 -> [w1277] mode=indexing
                tunnel: w1087 -> [w1273] mode=indexing
                shift-right: [w1269] -> _
                shift-left: dbl[] [] -> [w1272]
                shift-right: [w1267] -> w1170
                shift-left: dbl[][] [] -> [w1266]
                n869 = Index Array(array=w1272, index #1=0 ("index"), index #2=1 ("index")) -> (element #1=w1278:dbl, element #2=w1276:dbl)
                n870 = Add(x=w1277, y=w1278) -> (x+y=w1275:dbl)
                n871 = Add(x=w1276, y=w1273) -> (x+y=w1274:dbl)
                n872 = Build Array(w1275, w1274) -> (w1269:dbl[])
                n873 = Equal?(x=w1272, y=w1269) -> (x = y?=w1271:bool[])
                n874 = Insert Into Array(array=w1266, new element=w1269) -> (w1268:dbl[][])  [unwired: 2 in]
                n875 = And Array Elements(Boolean array=w1271) -> (logical AND=w1270:bool)
                n876 = Select(t=w1266, s=w1270, f=w1268) -> (s? t:f=w1267:dbl[][])
              }
              n877 = for {
                N -> [w1281]
                tunnel: w1111 -> [w1286] mode=indexing
                tunnel: w1113 -> [w1285] mode=indexing
                tunnel: [w1282] -> w1167 mode=indexing
                shift-right: [w1282] -> _
                shift-left: i64 0 -> [w1283]
                tunnel: [w1281] -> _ mode=indexing
                n878 = Subtract(x=w1286, y=w1285) -> (x-y=w1284:i64)
                n879 = Add(x=w1283, y=w1284) -> (x+y=w1282:i64)
              }
              n880 = Divide(x=w1167, y=i64 25 ("new element/subarray")) -> (x/y=w1166:dbl[])
              n881 = Index Array(array=w1175, index (col) #1=31 ("disabled index (col)"), index (col) #2=32 ("index (col)"), index (col) #3=33 ("index (col)"), index (col) #4=34 ("index (col)"), index (col) #5=0 ("index (col)")) -> (element #1=w1150:i64[], element #2=w1106:i64[], element #3=w1105:i64[], element #4=w1104:i64[], element #5=w1101:i64[])  [unwired: 5 in]
              n882 = Insert Into Array(array=w1099, index=w1164, new element=w1164) -> (w1132:dbl[])
              n883 = Insert Into Array(array=w1166, index=w1163, new element=w1163) -> (w1118:dbl[])
              n884 = Insert Into Array(array=w1098, index=w1165, new element=w1165) -> (w1133:dbl[])
              n885 = Insert Into Array(array=w1170, index (row)=0, new element=dbl[] [0.0, 0.0] ("new element/subarray")) -> (w1131:dbl[][])  [unwired: 1 in]
              n886 = for {
                tunnel: w1150 -> [w1265] mode=indexing
                tunnel: w1101 -> [w1263] mode=indexing
                tunnel: [w1263] -> w1110 mode=indexing if=w1264
                tunnel: [w1263] -> w1109 mode=indexing if=w1256
                tunnel: [w1263] -> w1108 mode=indexing if=w1257
                tunnel: [w1263] -> w1107 mode=indexing if=w1258
                tunnel: w1106 -> [w1262] mode=indexing
                tunnel: w1105 -> [w1261] mode=indexing
                tunnel: w1104 -> [w1260] mode=indexing
                w1259 = 1 ("x")
                n887 = Equal?(x=w1259, y=w1265) -> (x = y?=w1264:bool)
                n888 = Equal?(x=w1259, y=w1262) -> (x = y?=w1256:bool)
                n889 = Equal?(x=w1259, y=w1261) -> (x = y?=w1257:bool)
                n890 = Equal?(x=w1259, y=w1260) -> (x = y?=w1258:bool)
              }
              n891 = property on="momentum graph" class="XYGraph (strict)"() -> ("Cursor.Cursor X"=w1173:dbl)  [unwired: 2 in, 2 out]
              n892 = Search 1D Array(1D array=w1118, element=w1173) -> (index of element=w1123:i32)  [unwired: 1 in]
              n893 = for {
                tunnel: w1110 -> [w1255] mode=indexing
                tunnel: w1111 -> [w1254]
                tunnel: [w1252] -> w1148 mode=indexing
                tunnel: [w1249] -> w1149 mode=indexing
                tunnel: w1118 -> [w1248]
                tunnel: w1133 -> [w1247]
                n894 = Search 1D Array(1D array=w1254, element=w1255) -> (index of element=w1250:i32)  [unwired: 1 in]
                n895 = Increment(x=w1250) -> (x+1=w1253:i32)
                n896 = Increment(x=w1250) -> (x+1=w1251:i32)
                n897 = Index Array(array=w1248, index=w1253) -> (element=w1252:dbl)
                n898 = Index Array(array=w1247, index=w1251) -> (element=w1249:dbl)
              }
              n899 = for {
                tunnel: w1108 -> [w1237] mode=indexing
                tunnel: w1111 -> [w1236]
                tunnel: [w1234] -> w1143 mode=indexing
                tunnel: [w1231] -> w1142 mode=indexing
                tunnel: w1118 -> [w1230]
                tunnel: w1132 -> [w1229]
                n900 = Search 1D Array(1D array=w1236, element=w1237) -> (index of element=w1232:i32)  [unwired: 1 in]
                n901 = Increment(x=w1232) -> (x+1=w1235:i32)
                n902 = Increment(x=w1232) -> (x+1=w1233:i32)
                n903 = Index Array(array=w1230, index=w1235) -> (element=w1234:dbl)
                n904 = Index Array(array=w1229, index=w1233) -> (element=w1231:dbl)
              }
              n905 = for {
                tunnel: w1107 -> [w1228] mode=indexing
                tunnel: w1111 -> [w1227]
                tunnel: [w1225] -> w1141 mode=indexing
                tunnel: [w1222] -> w1140 mode=indexing
                tunnel: w1118 -> [w1221]
                tunnel: w1133 -> [w1220]
                n906 = Search 1D Array(1D array=w1227, element=w1228) -> (index of element=w1223:i32)  [unwired: 1 in]
                n907 = Increment(x=w1223) -> (x+1=w1226:i32)
                n908 = Increment(x=w1223) -> (x+1=w1224:i32)
                n909 = Index Array(array=w1221, index=w1226) -> (element=w1225:dbl)
                n910 = Index Array(array=w1220, index=w1224) -> (element=w1222:dbl)
              }
              n911 = for {
                tunnel: w1109 -> [w1246] mode=indexing
                tunnel: w1111 -> [w1245]
                tunnel: [w1243] -> w1151 mode=indexing
                tunnel: [w1240] -> w1152 mode=indexing
                tunnel: w1118 -> [w1239]
                tunnel: w1132 -> [w1238]
                n912 = Search 1D Array(1D array=w1245, element=w1246) -> (index of element=w1241:i32)  [unwired: 1 in]
                n913 = Increment(x=w1241) -> (x+1=w1244:i32)
                n914 = Increment(x=w1241) -> (x+1=w1242:i32)
                n915 = Index Array(array=w1239, index=w1244) -> (element=w1243:dbl)
                n916 = Index Array(array=w1238, index=w1242) -> (element=w1240:dbl)
              }
              n917 = Decrement(x=w1123) -> (x-1=w1124:i32)
              n918 = Index Array(array=w1131, index (row)=w1123) -> (element=→"Score":dbl[])  [unwired: 1 in]
              n919 = Array Max & Min(array=w1118) -> (max value=w1127:dbl)  [unwired: 3 out]
              n920 = Array Size(array=w1131) -> (size(s)=w1130:i32[])
              n921 = Index Array(array=w1118, index #1=w1123, index #2=w1124) -> (element #1=w1121:dbl, element #2=w1122:dbl)
              n922 = Delete From Array(array=w1118, index=0) -> (array with subset deleted=w1117:dbl[])  [unwired: 1 in, 1 out]
              n923 = Index Array(array=w1130, index=0) -> (element=w1128:i32)
              n924 = Subtract(x=w1121, y=w1122) -> (x-y=→"Rally length(sec)":dbl)
              n925 = Subtract(x=w1117, y=w1118) -> (x-y=w1116:dbl[])
              n926 = Decrement(x=w1128) -> (x-1=w1126:i32)
              n927 = Array Max & Min(array=w1116) -> (max value=→"Longest rally length(sec)":dbl, min value=→"Shortest rally length(sec)":dbl)  [unwired: 2 out]
              n928 = Bundle(w1118, w1132) -> (w1160:cluster{dbl[], dbl[]})  [unwired: 1 in]
              n929 = Bundle(w1141, w1140) -> (w1136:cluster{dbl[], dbl[]})  [unwired: 1 in]
              n930 = Bundle(w1118, w1133) -> (w1161:cluster{dbl[], dbl[]})  [unwired: 1 in]
              n931 = Bundle(w1151, w1152) -> (w1138:cluster{dbl[], dbl[]})  [unwired: 1 in]
              n932 = Bundle(w1143, w1142) -> (w1137:cluster{dbl[], dbl[]})  [unwired: 1 in]
              n933 = Bundle(w1148, w1149) -> (w1139:cluster{dbl[], dbl[]})  [unwired: 1 in]
              n934 = Divide(x=w1127, y=w1126) -> (x/y=→"Average rally length(sec)":dbl)
              n935 = Build Array(w1139, w1138, w1137, w1136, w1161, w1160) -> (→"momentum graph":cluster{dbl[], dbl[]}[])
              n936 = local read "Video files to write"() -> (w1093:string[])
              n937 = property on="Video files to write" class="Arr (strict)"() -> ("Index Values"=w1092:u32[])  [unwired: 2 in, 2 out]
              n938 = local read "frames to write"() -> (w1094:i64[][])
              n939 = case shown="True" "Upload edited video" {
                frame False {
                }
                frame True {
                  n940 = flat-sequence {
                    frame #0 {
                      n941 = local read "frames edited"() -> (w1197:i64[])
                      n942 = local write "Progress..."(u32 0 ("Progress...")) -> ()
                      n943 = local write "frames 2 play"(w1197) -> ()
                    }
                    frame #1 {
                      w1199 = FALSE ("stop")
                      w1200 = TRUE ("Play")
                      n944 = local write "Load video"(w1200) -> ()
                      n945 = local write "Play"(w1200) -> ()
                      n946 = local write "stop"(w1199) -> ()
                      n947 = local write "Upload edited video"(w1199) -> ()
                      n948 = local write "Pause"(w1199) -> ()
                    }
                  }
                }
              }
              n949 = Index Array(array=w1092) -> (element=w1089:u32)  [unwired: 1 in]
              n950 = And Array Elements(Boolean array="Delete") -> (logical AND=w1091:bool)
              n951 = case shown="True" "Add to lib" {
                tunnel: w1094 -> [_ w1192]
                tunnel: w1093 -> [_ w1189]
                frame False {
                }
                frame True {
                  n952 = local read "frames edited"() -> (w1188:i64[])
                  n953 = local write "Add to lib"(FALSE ("Add to lib")) -> ()
                  n954 = Build Array("File name") -> (w1190:string[])
                  n955 = Build Array(w1188) -> (w1193:i64[][])
                  n956 = Insert Into Array(array=w1193, new element=w1192) -> (→"frames to write":i64[][])  [unwired: 2 in]
                  n957 = Insert Into Array(array=w1190, new element=w1189) -> (→"Video files to write":string[])  [unwired: 1 in]
                }
              }
              n958 = case shown="False" w1091 {
                tunnel: "Delete" -> [w1184 _]
                tunnel: w1089 -> [w1182 _]
                frame False {
                  n959 = for {
                    tunnel: w1184 -> [w1187] mode=indexing
                    tunnel: [w1185] -> w1183
                    i -> [w1185]
                    stop <- w1186 stop-if-true
                    n960 = Not(x=w1187) -> (.not. x?=w1186:bool)
                  }
                  n961 = local write "Delete"(bool[] [TRUE, TRUE, TRUE, TRUE, TRUE] ("Array 2")) -> ()
                  n962 = local read "Video files to write"() -> (w1179:string[])
                  n963 = local read "frames to write"() -> (w1177:i64[][])
                  n964 = Add(x=w1183, y=w1182) -> (x+y=w1176:u32)
                  n965 = Delete From Array(array=w1179, index=w1176) -> (array with subset deleted=w1181:string[])  [unwired: 1 in, 1 out]
                  n966 = Delete From Array(array=w1177, index (row)=w1176) -> (array with subset deleted=w1178:i64[][])  [unwired: 2 in, 1 out]
                  n967 = local write "frames to write"(w1178) -> ()
                  n968 = local write "Video files to write"(w1181) -> ()
                }
                frame True {
                }
              }
            }
            frame #1 {
              w1297 = dbl[] [0.0, 0.0, 0.0, 0.0, 0.0, 0.0, 0.0, 0.0, 0.0, 0.0, 0.0] ("array")
              w1311 = "" ("new element/subarray")
              w1339 = "" ("new element/subarray")
              w1349 = string[] ["Winners", "Errors"] ("W/E1")
              w1350 = string[] ["Fore hand", "Back hand", "Over head", "", "Straight", "Cross", "", "Smash", "Half smash", "DRIVE DEF", "BLOCK DEF", "CLEAR DEF", "Drive/Tap", "Lob", "Drop", "Clear", "Net"] ("Player 2")
              w1294 = 0.0 ("X Scale.Range:Minimum")
              w1466 = i16 1 ("width (-)")
              w1517 = 15 ("index")
              w1512 = 15 ("index")
              n969 = local read "edited\nevents"() -> (w1487:i64[][])
              n970 = local read "Compare"() -> (w1443:bool)
              n971 = case shown="\"4\"" "2 8" {
                tunnel: [w1566 w1567 w1568] -> w1475
                frame "1", Default {
                  n972 = local read "game"() -> (w1566:i32[][])
                }
                frame "3" {
                  n973 = local read "save1 2"() -> (w1567:i32[][])
                }
                frame "4" {
                  n974 = local read "save2 2"() -> (w1568:i32[][])
                }
              }
              n975 = case shown="\"1\", Default" "1 8" {
                tunnel: [w1569 w1570 w1571] -> w1479
                frame "1", Default {
                  n976 = local read "game"() -> (w1569:i32[][])
                }
                frame "3" {
                  n977 = local read "save1 2"() -> (w1570:i32[][])
                }
                frame "4" {
                  n978 = local read "save2 2"() -> (w1571:i32[][])
                }
              }
              n979 = case shown="False" w1443 {
                frame False {
                  w1560 = u8 0 ("Disabled")
                  n980 = local read "Percentage"() -> (w1561:bool)
                  n981 = local write "Percentage"(w1561) -> ()
                  n982 = local read "display\nselection"() -> (w1562:string)
                  n983 = local write "display\nselection"(w1562) -> ()
                  n984 = property on="display\nselection" class="CmbBox"("Disabled"=w1560) -> ()  [unwired: 2 in, 2 out]
                  n985 = property on="Percentage" class="Bool (strict)"("Disabled"=w1560) -> ()  [unwired: 2 in, 2 out]
                }
                frame True {
                  w1563 = u8 2 ("Disabled")
                  n986 = local read "1 8"() -> (w1565:string)
                  n987 = local write "display\nselection"(w1565) -> ()
                  n988 = property on="display\nselection" class="CmbBox"("Disabled"=w1563) -> ()  [unwired: 2 in, 2 out]
                  n989 = property on="Percentage" class="Bool (strict)"("Disabled"=w1563) -> ()  [unwired: 2 in, 2 out]
                  n990 = local write "Percentage"(TRUE ("t")) -> ()
                }
              }
              n991 = Index Array(array=w1414, index (col)=0 ("disabled index (col)")) -> (element=w1494:i64[])  [unwired: 1 in]
              n992 = Index Array(array=w1487, index (col)=0 ("disabled index (col)")) -> (element=w1492:i64[])  [unwired: 1 in]
              n993 = for {
                tunnel: w1494 -> [w1587]
                tunnel: w1492 -> [w1586] mode=indexing
                tunnel: [w1584] -> w1485 mode=indexing
                tunnel: w1414 -> [w1583]
                i -> [w1588]
                n994 = Search 1D Array(1D array=w1587, element=w1586, start index (0)=w1588) -> (index of element=w1585:i32)
                n995 = Index Array(array=w1583, index (row)=w1585) -> (element=w1584:i64[])  [unwired: 1 in]
              }
              n996 = Index Array(array=w1475, index (row) #1=0 ("index (row)"), index (row) #2=1 ("index (row)")) -> (element #1=w1473:i32[], element #2=w1471:i32[])  [unwired: 2 in]
              n997 = Index Array(array=w1479, index (row) #1=0 ("index (row)"), index (row) #2=1 ("index (row)")) -> (element #1=w1474:i32[], element #2=w1472:i32[])  [unwired: 2 in]
              n998 = Divide(x=w1474, y=w1473) -> (x/y=w1468:dbl[])
              n999 = Divide(x=w1472, y=w1471) -> (x/y=w1467:dbl[])
              n1000 = Multiply(x=w1467, y=100.0 ("new element/subarray")) -> (x*y=w1462:dbl[])
              n1001 = Multiply(x=100.0 ("new element/subarray"), y=w1468) -> (x*y=w1465:dbl[])
              n1002 = Split 1D Array(array=w1465, index=30) -> (first subarray=→"comp_p1":dbl[], second subarray=→"comp_p1 2":dbl[])
              n1003 = Split 1D Array(array=w1462, index=30) -> (first subarray=→"comp_p2":dbl[], second subarray=→"comp_p2 2":dbl[])
              n1004 = case shown="\"1\", Default" "display\nselection" {
                tunnel: [w1573 w1574 w1575 w1576] -> w1486
                tunnel: w1485 -> [_ w1574 _ _]
                tunnel: w1414 -> [w1573 _ _ _]
                frame "1", Default {
                }
                frame "2" {
                }
                frame "3" {
                  n1005 = local read "save1_data"() -> (w1575:dbl[][])
                }
                frame "4" {
                  n1006 = local read "save2_data"() -> (w1576:dbl[][])
                }
              }
              n1007 = Index Array(array=w1486, index (col) #1=48 ("disabled index (col)"), index (col) #2=49 ("index (col)")) -> (element #1=w1502:dbl[], element #2=w1499:dbl[])  [unwired: 2 in]
              n1008 = for {
                N: 30 -> [_]
                tunnel: w1486 -> [w1623]
                tunnel: w1502 -> [w1622]
                tunnel: w1499 -> [w1621]
                tunnel: [w1619] -> w1500 mode=indexing
                tunnel: [w1618] -> w1501 mode=indexing
                i -> [w1616]
                n1009 = Increment(x=w1616) -> (x+1=w1617:i32)
                n1010 = Index Array(array=w1623, index (col)=w1617) -> (element=w1620:dbl[])  [unwired: 1 in]
                n1011 = And(x=w1622, y=w1620) -> (x .and. y?=w1619:i32[])
                n1012 = And(x=w1621, y=w1620) -> (x .and. y?=w1618:i32[])
              }
              n1013 = Index Array(array=w1486, index (col) #1=31 ("disabled index (col)"), index (col) #2=33 ("index (col)"), index (col) #3=32 ("index (col)"), index (col) #4=34 ("index (col)")) -> (element #1=w1545:dbl[], element #2=w1550:dbl[], element #3=w1551:dbl[], element #4=w1549:dbl[])  [unwired: 4 in]
              n1014 = Add Array Elements(numeric array=w1545) -> (sum=w1554:dbl)
              n1015 = Add Array Elements(numeric array=w1551) -> (sum=w1553:dbl)
              n1016 = local read "comp_p1 2"() -> (w1441:dbl[])
              n1017 = local read "Compare"() -> (w1453:bool)
              n1018 = local read "comp_p2 2"() -> (w1449:dbl[])
              n1019 = Add Array Elements(numeric array=w1549) -> (sum=w1552:dbl)
              n1020 = Add Array Elements(numeric array=w1550) -> (sum=w1555:dbl)
              n1021 = local read "Compare"() -> (w1450:bool)
              n1022 = Build Array(w1554, w1555) -> (w1452:dbl[])
              n1023 = Build Array(w1553, w1552) -> (w1442:dbl[])
              n1024 = Transpose 2D Array(2D array=w1500) -> (transposed array=w1511:i32[][])
              n1025 = Transpose 2D Array(2D array=w1501) -> (transposed array=w1510:i32[][])
              n1026 = Select(t=w1441, s=w1453, f=w1452) -> (s? t:f=w1451:dbl[])
              n1027 = Select(t=w1449, s=w1450, f=w1442) -> (s? t:f=w1448:dbl[])
              n1028 = for {
                N: 30 -> [_]
                tunnel: w1511 -> [w1615]
                tunnel: w1510 -> [w1614]
                tunnel: [w1611] -> w1417 mode=indexing
                tunnel: [w1610] -> w1413 mode=indexing
                i -> [w1613]
                n1029 = Index Array(array=w1615, index (col)=w1613) -> (element=w1612:i32[])  [unwired: 1 in]
                n1030 = Index Array(array=w1614, index (col)=w1613) -> (element=w1609:i32[])  [unwired: 1 in]
                n1031 = Add Array Elements(numeric array=w1612) -> (sum=w1611:i32)
                n1032 = Add Array Elements(numeric array=w1609) -> (sum=w1610:i32)
              }
              n1033 = Number To Decimal String(number=w1451, width (-)=w1466) -> (decimal integer string=→"W1/E1":string[])
              n1034 = Number To Decimal String(number=w1448, width (-)=w1466) -> (decimal integer string=→"W2/E2":string[])
              n1035 = Split 1D Array(array=w1417, index=w1512) -> (first subarray=w1513:i32[], second subarray=w1415:i32[])
              n1036 = Split 1D Array(array=w1413, index=w1517) -> (first subarray=w1516:i32[], second subarray=w1521:i32[])
              n1037 = Insert Into Array(array=w1417, new element=w1441) -> (w1491:i32[])  [unwired: 1 in]
              n1038 = Insert Into Array(array=w1413, new element=w1442) -> (w1490:i32[])  [unwired: 1 in]
              n1039 = Add Array Elements(numeric array=w1516) -> (sum=w1515:i32)
              n1040 = Add Array Elements(numeric array=w1513) -> (sum=w1514:i32)
              n1041 = Build Array(w1491, w1490) -> (w1483:i32[][])
              n1042 = Index Array(array=w1521, index #1=3 ("index"), index #2=4 ("index")) -> (element #1=w1509:i32, element #2=w1508:i32)
              n1043 = Index Array(array=w1415, index #1=3 ("index"), index #2=4 ("index")) -> (element #1=w1518:i32, element #2=w1519:i32)
              n1044 = for {
                N: w1512 -> [_]
                tunnel: w1513 -> [w1608] mode=indexing
                tunnel: w1514 -> [w1607]
                tunnel: [w1604] -> w1523 mode=indexing
                n1045 = Divide(x=w1608, y=w1607) -> (x/y=w1606:dbl)
                n1046 = Multiply(x=w1606, y=100.0) -> (x*y=w1604:dbl)
              }
              n1047 = Add(x=w1509, y=w1508) -> (x+y=w1520:i32)
              n1048 = for {
                N: w1517 -> [_]
                tunnel: w1516 -> [w1603] mode=indexing
                tunnel: w1515 -> [w1602]
                tunnel: [w1599] -> w1445 mode=indexing
                n1049 = Divide(x=w1603, y=w1602) -> (x/y=w1601:dbl)
                n1050 = Multiply(x=w1601, y=100.0) -> (x*y=w1599:dbl)
              }
              n1051 = Add(x=w1518, y=w1519) -> (x+y=w1522:i32)
              n1052 = case shown="\"1\"" "display\nselection" {
                tunnel: w1483 -> [_ w1572 _]
                frame "0", Default {
                }
                frame "1" {
                  "game" <- w1572
                }
                frame "2" {
                }
              }
              n1053 = case shown="True" "save2 3" {
                tunnel: w1483 -> [_ w1579]
                tunnel: w1486 -> [_ w1577]
                frame False {
                }
                frame True {
                  n1054 = local write "save2 3"(FALSE ("save2")) -> ()
                  "save2 2" <- w1579
                  "save2_data" <- w1577
                }
              }
              n1055 = case shown="True" "save1 3" {
                tunnel: w1483 -> [_ w1582]
                tunnel: w1486 -> [_ w1580]
                frame False {
                }
                frame True {
                  n1056 = local write "save1 3"(FALSE ("save1")) -> ()
                  "save1 2" <- w1582
                  "save1_data" <- w1580
                }
              }
              n1057 = for {
                tunnel: w1521 -> [w1598] mode=indexing
                tunnel: w1520 -> [w1597]
                tunnel: [w1594] -> w1525 mode=indexing
                n1058 = Divide(x=w1598, y=w1597) -> (x/y=w1596:dbl)
                n1059 = Multiply(x=w1596, y=100.0) -> (x*y=w1594:dbl)
              }
              n1060 = for {
                tunnel: w1415 -> [w1593] mode=indexing
                tunnel: w1522 -> [w1592]
                tunnel: [w1589] -> w1524 mode=indexing
                n1061 = Divide(x=w1593, y=w1592) -> (x/y=w1591:dbl)
                n1062 = Multiply(x=w1591, y=100.0) -> (x*y=w1589:dbl)
              }
              n1063 = local read "comp_p2"() -> (w1457:dbl[])
              n1064 = local read "Compare"() -> (w1456:bool)
              n1065 = local read "comp_p1"() -> (w1458:dbl[])
              n1066 = Insert Into Array(array=w1445, new element=w1525) -> (w1444:dbl[])  [unwired: 1 in]
              n1067 = Insert Into Array(array=w1523, new element=w1524) -> (w1446:dbl[])  [unwired: 1 in]
              n1068 = Select(t=w1457, s=w1456, f=w1444) -> (s? t:f=w1426:dbl[])
              n1069 = Select(t=w1458, s="Compare", f=w1446) -> (s? t:f=w1421:dbl[])
              n1070 = local read "Percentage"() -> (w1542:bool)
              n1071 = local read "Percentage"() -> (w1543:bool)
              n1072 = Split 1D Array(array=w1426, index=15) -> (second subarray=w1531:dbl[])  [unwired: 1 out]
              n1073 = Number To Fractional String(number=w1426, precision (6)=i16 0) -> (F-format string=w1425:string[])  [unwired: 2 in]
              n1074 = Split 1D Array(array=w1413, index=15) -> (second subarray=w1534:i32[])  [unwired: 1 out]
              n1075 = Split 1D Array(array=w1421, index=15) -> (second subarray=w1530:dbl[])  [unwired: 1 out]
              n1076 = Number To Fractional String(number=w1421, precision (6)=i16 0) -> (F-format string=w1418:string[])  [unwired: 2 in]
              n1077 = Split 1D Array(array=w1417, index=15) -> (second subarray=w1528:i32[])  [unwired: 1 out]
              n1078 = local read "Percentage"() -> (w1538:bool)
              n1079 = Number To Fractional String(number=w1417, precision (6)=i16 0) -> (F-format string=w1419:string[])  [unwired: 2 in]
              n1080 = Number To Decimal String(number=w1528, width (-)=i16 1 ("precision (6)")) -> (decimal integer string=w1537:string[])
              n1081 = Number To Fractional String(number=w1413, precision (6)=i16 0) -> (F-format string=w1423:string[])  [unwired: 2 in]
              n1082 = Number To Fractional String(number=w1530, precision (6)=i16 0) -> (F-format string=w1536:string[])  [unwired: 2 in]
              n1083 = Number To Decimal String(number=w1534, width (-)=i16 1 ("precision (6)")) -> (decimal integer string=w1540:string[])
              n1084 = Number To Fractional String(number=w1531, precision (6)=i16 0) -> (F-format string=w1539:string[])  [unwired: 2 in]
              n1085 = Select(t=w1418, s=w1543, f=w1419) -> (s? t:f=w1416:string[])
              n1086 = Select(t=w1536, s="Percentage", f=w1537) -> (s? t:f=w1431:string[])
              n1087 = call "Search NaN_Inf (SubVI).vi"("in"=w1416) -> ("out"=w1382:string[])
              n1088 = Select(t=w1539, s=w1538, f=w1540) -> (s? t:f=w1430:string[])
              n1089 = Select(t=w1425, s=w1542, f=w1423) -> (s? t:f=w1427:string[])
              n1090 = call "Search NaN_Inf (SubVI).vi"("in"=w1431) -> ("out"=w1303:string[])
              n1091 = call "Search NaN_Inf (SubVI).vi"("in"=w1427) -> ("out"=w1351:string[])
              n1092 = call "Search NaN_Inf (SubVI).vi"("in"=w1430) -> ("out"=w1326:string[])
              n1093 = Insert Into Array(array=w1303, index=3, new element=w1311) -> (w1309:string[])
              n1094 = Insert Into Array(array=w1326, index=3, new element=w1339) -> (w1341:string[])
              n1095 = Insert Into Array(array=w1309, index=6, new element=w1311) -> (w1304:string[])
              n1096 = Index Array(array=w1382, index #1=0 ("index"), index #2=1 ("index"), index #3=2 ("index"), index #4=3 ("index"), index #5=4 ("index"), index #6=5 ("index"), index #7=6 ("index"), index #8=7 ("index"), index #9=8 ("index"), index #10=9 ("index"), index #11=10 ("index"), index #12=11 ("index"), index #13=12 ("index"), index #14=13 ("index"), index #15=14 ("index")) -> (element #1=→"p1 1":string, element #2=→"p1 2":string, element #3=→"p1 3":string, element #4=→"p1 4":string, element #5=→"p1 5":string, element #6=→"p1 6":string, element #7=→"p1 7":string, element #8=→"p1 8":string, element #9=→"p1 9":string, element #10=→"p1 10":string, element #11=→"p1 11":string, element #12=→"p1 12":string, element #13=→"p1 13":string, element #14=→"p1 14":string, element #15=→"p1 15":string)
              n1097 = Insert Into Array(array=w1341, index=6, new element=w1339) -> (w1346:string[])
              n1098 = Index Array(array=w1351, index #1=0 ("index"), index #2=1 ("index"), index #3=2 ("index"), index #4=3 ("index"), index #5=4 ("index"), index #6=5 ("index"), index #7=6 ("index"), index #8=7 ("index"), index #9=8 ("index"), index #10=9 ("index"), index #11=10 ("index"), index #12=11 ("index"), index #13=12 ("index"), index #14=13 ("index"), index #15=14 ("index")) -> (element #1=→"p2 17":string, element #2=→"p2 16":string, element #3=→"p2 12":string, element #4=→"p2 13":string, element #5=→"p2 15":string, element #6=→"p2 14":string, element #7=→"p2 10":string, element #8=→"p2 11":string, element #9=→"p2 9":string, element #10=→"p2 18":string, element #11=→"p2 19":string, element #12=→"p2 20":string, element #13=→"p2 21":string, element #14=→"p2 22":string, element #15=→"p2 23":string)
              n1099 = Split 1D Array(array=w1304, index=6) -> (first subarray=→"player1_2":string[], second subarray=w1306:string[])
              n1100 = Split 1D Array(array=w1346, index=6) -> (first subarray=→"player2_2":string[], second subarray=w1344:string[])
              n1101 = Delete From Array(array=w1306, index=0) -> (array with subset deleted=w1323:string[])  [unwired: 1 in, 1 out]
              n1102 = Delete From Array(array=w1344, index=0) -> (array with subset deleted=w1327:string[])  [unwired: 1 in, 1 out]
              n1103 = Delete From Array(array=w1323, length=2, index=8) -> (deleted portion=w1321:string[], array with subset deleted=w1312:string[])
              n1104 = Delete From Array(array=w1327, length=2, index=8) -> (deleted portion=w1329:string[], array with subset deleted=w1338:string[])
              n1105 = Delete From Array(array=w1312, length=1, index=5) -> (deleted portion=w1318:string[], array with subset deleted=w1317:string[])
              n1106 = Delete From Array(array=w1338, length=1, index=5) -> (deleted portion=w1332:string[], array with subset deleted=w1333:string[])
              n1107 = Insert Into Array(array=w1317, index=1, new element=w1318) -> (w1320:string[])
              n1108 = Insert Into Array(array=w1333, index=1, new element=w1332) -> (w1330:string[])
              n1109 = Insert Into Array(array=w1320, index=3, new element=w1321) -> (w1301:string[])
              "player1 2" <- w1301
              n1110 = Insert Into Array(array=w1330, index=3, new element=w1329) -> (w1324:string[])
              "player2 2" <- w1324
              n1111 = Fract/Exp String To Number(string=w1301) -> (number=w1302:dbl[])  [unwired: 3 in, 1 out]
              n1112 = Fract/Exp String To Number(string=w1324) -> (number=w1429:dbl[])  [unwired: 3 in, 1 out]
              n1113 = Array Max & Min(array=w1302) -> (max value=w1438:dbl)  [unwired: 3 out]
              n1114 = Array Max & Min(array=w1429) -> (max value=w1437:dbl)  [unwired: 3 out]
              n1115 = Interleave 1D Arrays(w1297, w1302) -> (w1440:dbl[])
              n1116 = Insert Into Array(array=w1440, new element=0.0 ("new element/subarray")) -> (w1557:dbl[])  [unwired: 1 in]
              n1117 = Max & Min(x=w1438, y=w1437) -> (max(x,y)=w1432:dbl)  [unwired: 1 out]
              n1118 = Interleave 1D Arrays(w1297, w1429) -> (w1439:dbl[])
              n1119 = Bundle(w1557, "array"=dbl[] [1.0, 2.0, 3.0, 4.0, 5.0, 6.0, 7.0, 8.0, 9.0, 10.0, 11.0, 12.0, 13.0, 14.0, 15.0, 16.0, 17.0, 18.0, 19.0, 20.0, 21.0]) -> (→"P1graph":cluster{dbl[], "array":dbl[]})  [unwired: 1 in]
              n1120 = Equal?(x=w1432, y=inf) -> (x = y?=w1434:bool)
              n1121 = Insert Into Array(array=w1439, new element=0.0 ("new element/subarray")) -> (w1558:dbl[])  [unwired: 1 in]
              n1122 = Select(t=100.0, s=w1434, f=w1432) -> (s? t:f=w1295:dbl)
              n1123 = Bundle(w1558, "array"=dbl[] [1.0, 2.0, 3.0, 4.0, 5.0, 6.0, 7.0, 8.0, 9.0, 10.0, 11.0, 12.0, 13.0, 14.0, 15.0, 16.0, 17.0, 18.0, 19.0, 20.0, 21.0]) -> (→"P2graph":cluster{dbl[], "array":dbl[]})  [unwired: 1 in]
              n1124 = property on="P1graph" class="XYGraph (strict)"("XScale.Maximum"=w1295, "XScale.Minimum"=w1294) -> ()  [unwired: 2 in, 2 out]
              n1125 = property on="P2graph" class="XYGraph (strict)"("XScale.Maximum"=w1295, "XScale.Minimum"=w1294) -> ()  [unwired: 2 in, 2 out]
              "Player 6" <- w1350
              "Player 1_2" <- w1350
              "Player 2_2" <- w1350
              "Player 5" <- w1350
              "W/E1" <- w1349
              "W/E2" <- w1349
            }
          }
          n1126 = local read "refnum of data save file"() -> (w1073:refnum<file>)
          n1127 = local write "Code number"(0 ("Code number")) -> ()
          n1128 = Select(t=T2."Edit video" ("Main tab"), s="Extract data", f=T2."Display" ("Main tab")) -> (s? t:f=w1081:T2)
          n1129 = Select(t=T2."Examine coding" ("Main tab"), s="Examine code", f=w1081) -> (s? t:f=w1082:T2)
        }
        frame "Edit video" {
          n1130 = Build Array("TL", "TCL", "TC", "TCR", "TR", "ML", "MCL", "MC", "MCR", "MR", "BL", "BCL", "BC", "BCR", "BR", "FH 2", "BH 2", "OH 2", "ST", "CR 2", "smash", "Dr def", "drive", "lob", "drop", "Hf smash", "clear", "net", "Blk def", "clear def", "winner", "winner", "error", "error", "point 1", "point 2", "service1", "service2", "service3", "service4", "1 9", "2 9", "3 8", "4 8", "5 8", "Team 1", "Team 2", "player1", "player2", "player3", "player4") -> (w1625:bool[])
          "Last Edit" <- w1625
          n1131 = Delete From Array(array=w1624, length=2, index (col)=37 ("disabled index (col)")) -> (deleted portion=→"Score 2":i64[][], array with subset deleted=w1688:i64[][])  [unwired: 1 in]
          n1132 = Index Array(array=w1688, index (col) #1=31 ("disabled index (col)"), index (col) #2=32 ("index (col)"), index (col) #3=33 ("index (col)"), index (col) #4=34 ("index (col)")) -> (element #1=w1698:i64[], element #2=w1697:i64[], element #3=w1696:i64[], element #4=w1695:i64[])  [unwired: 4 in]
          n1133 = Or(x=w1696, y=w1695) -> (x .or. y?=w1689:i64[])
          n1134 = Or(x=w1698, y=w1697) -> (x .or. y?=w1694:i64[])
          n1135 = Replace Array Subset(array=w1688, new element #1=w1694, index (col) #1=31 ("disabled index (col)"), new element #2=w1694, index (col) #2=32 ("index (col)"), new element #3=w1689, index (col) #3=33 ("index (col)"), new element #4=w1689, index (col) #4=34 ("index (col)")) -> (w1687:i64[][])  [unwired: 4 in]
          n1136 = Delete From Array(array=w1687, length=1, index (col)=0 ("disabled index (col)")) -> (deleted portion=w1685:i64[][], array with subset deleted=w1686:i64[][])  [unwired: 1 in]
          "frame data" <- w1685
          "coded data" <- w1686
          n1137 = Or Array Elements(Boolean array=w1625) -> (logical OR=w1684:bool)
          n1138 = case shown="True" w1684 {
            tunnel: w1686 -> [_ w1752]
            tunnel: w1625 -> [_ w1748]
            tunnel: w1685 -> [w1726 w1747]
            tunnel: [w1729 w1735] -> w1678
            frame False {
              n1139 = Delete From Array(array=w1726, length=1, index (col)=0 ("disabled index (col)")) -> (deleted portion=w1725:i64[][])  [unwired: 1 in, 1 out]
              n1140 = Array Max & Min(array=w1725) -> (max value=w1727:i64, min value=w1728:i64)  [unwired: 2 out]
              n1141 = for {
                N: 300 -> [_]
                i -> [w1733]
                n1142 = Increment(x=w1733) -> (x+1=w1732:i32)
                n1143 = local write "task"(w1732) -> ()
                n1144 = Wait (ms)(milliseconds to wait=u32 1) -> ()  [unwired: 1 out]
              }
              n1145 = Build Array(w1728, w1727) -> (w1729:i64[])
            }
            frame True {
              n1146 = for {
                tunnel: w1748 -> [w1782] mode=indexing
                tunnel: w1752 -> [w1785]
                tunnel: [w1783] -> w1737 mode=indexing if=w1782
                i -> [w1784]
                n1147 = Index Array(array=w1785, index (col)=w1784) -> (element=w1783:i64[])  [unwired: 1 in]
              }
              n1148 = Transpose 2D Array(2D array=w1737) -> (transposed array=w1751:i64[][])
              n1149 = for {
                tunnel: w1747 -> [w1779] mode=indexing
                tunnel: w1751 -> [w1777] mode=indexing
                tunnel: [w1778] -> w1750 mode=indexing
                tunnel: [w1779] -> w1736 mode=indexing if=w1778
                n1150 = Array Max & Min(array=w1777) -> (min value=w1780:i64)  [unwired: 3 out]
                n1151 = Equal?(x=w1780, y=1) -> (x = y?=w1778:bool)
              }
              "edited\nevents" <- w1736
              n1152 = Or Array Elements(Boolean array=w1750) -> (logical OR=w1749:bool)
              n1153 = Multiply(x="before", y=u32 25) -> (x*y=w1743:u32)
              n1154 = Multiply(x="after", y=u32 25) -> (x*y=w1744:u32)
              n1155 = Index Array(array=w1736, index (col)=0 ("disabled index (col)")) -> (element=w1746:i64[])  [unwired: 1 in]
              n1156 = for {
                tunnel: w1743 -> [w1762]
                tunnel: w1744 -> [w1764]
                tunnel: w1746 -> [w1763] mode=indexing
                shift-right: [w1756] -> w1735
                shift-left: u32[] [] -> [w1758]
                n1157 = Subtract(x=w1763, y=w1762) -> (x-y=w1760:i64)
                n1158 = Add(x=w1764, y=w1763) -> (x+y=w1759:i64)
                n1159 = Array Max & Min(array=w1758) -> (max value=w1761:u32, max index (indices)=w1757:i32)  [unwired: 2 out]
                n1160 = Greater Or Equal?(x=w1761, y=w1760) -> (x >= y?=w1755:bool)
                n1161 = Build Array(w1760, w1759) -> (w1753:i64[])
                n1162 = Build Array(w1759) -> (w1754:i64[])
                n1163 = case shown="True" w1755 {
                  tunnel: w1758 -> [w1767 w1771]
                  tunnel: w1757 -> [_ w1770]
                  tunnel: w1754 -> [_ w1769]
                  tunnel: [w1766 w1768] -> w1756
                  tunnel: w1753 -> [w1765 _]
                  frame False {
                    n1164 = Insert Into Array(array=w1767, new element=w1765) -> (w1766:u32[])  [unwired: 1 in]
                  }
                  frame True {
                    n1165 = Replace Array Subset(array=w1771, new element=w1769, index=w1770) -> (w1768:u32[])
                  }
                }
              }
              n1166 = case shown="False" w1749 {
                frame False {
                  n1167 = One Button Dialog(message="This combination \nof events are \nnot available") -> ()  [unwired: 1 in, 1 out]
                }
                frame True {
                  n1168 = for {
                    N: 300 -> [_]
                    i -> [w1775]
                    n1169 = Increment(x=w1775) -> (x+1=w1774:i32)
                    n1170 = local write "task"(w1774) -> ()
                    n1171 = Wait (ms)(milliseconds to wait=u32 1) -> ()  [unwired: 1 out]
                  }
                }
              }
            }
          }
          "edited to play" <- w1678
          n1172 = local write "Extract data"(FALSE ("edit video")) -> ()
          n1173 = Array Size(array=w1678) -> (size(s)=w1683:i32)
          n1174 = Divide(x=w1683, y=2) -> (x/y=w1682:dbl)
          n1175 = for {
            N: w1682 -> [_]
            shift-right: [w1714] -> _
            shift-left: w1678 -> [w1716]
            shift-right: [w1709] -> w1679
            shift-left: i64[] [] ("edited\nto play 3") -> [w1710]
            n1176 = Split 1D Array(array=w1716, index=2) -> (first subarray=w1715:i64[], second subarray=w1714:i64[])
            n1177 = Index Array(array=w1715, index #1=1 ("index"), index #2=0 ("index")) -> (element #1=w1720:i64, element #2=w1713:i64)
            n1178 = Subtract(x=w1720, y=w1713) -> (x-y=w1712:i64)
            n1179 = Increment(x=w1712) -> (x+1=w1711:i64)
            n1180 = for {
              N: w1711 -> [_]
              tunnel: w1713 -> [w1723]
              tunnel: [w1721] -> w1708 mode=indexing
              i -> [w1722]
              n1181 = Add(x=w1723, y=w1722) -> (x+y=w1721:i64)
            }
            n1182 = Insert Into Array(array=w1710, new element=w1708) -> (w1709:i64[])  [unwired: 1 in]
          }
          "frames edited" <- w1679
          "frames 2 play" <- w1679
          n1183 = local read "refnum of data save file"() -> (w1675:refnum<file>)
        }
        frame "Examine coding" {
          n1184 = local read "edited\nevents"() -> (w1846:i64[][])
          n1185 = Index Array(array=w1846, index (row)="Code number", index (col)=0) -> (element=w1845:i64)
          n1186 = Increment(x="Code number") -> (x+1=w1842:i32)
          "Code number display" <- w1842
          n1187 = flat-sequence {
            tunnel: w1842 -> [w1864]
            frame #0 {
              n1188 = local read "edited to play"() -> (w1863:i64[])
              n1189 = for {
                N: w1864 -> [_]
                shift-right: [w1869] -> _
                shift-left: w1863 -> [w1870]
                tunnel: [w1868] -> w1856
                n1190 = Split 1D Array(array=w1870, index=2) -> (first subarray=w1868:i64[], second subarray=w1869:i64[])
              }
              n1191 = Index Array(array=w1856, index #1=1 ("index"), index #2=0 ("index")) -> (element #1=w1862:i64, element #2=w1859:i64)
              n1192 = Subtract(x=w1862, y=w1859) -> (x-y=w1858:i64)
              n1193 = Increment(x=w1858) -> (x+1=w1857:i64)
              n1194 = for {
                N: w1857 -> [_]
                tunnel: w1859 -> [w1867]
                tunnel: [w1865] -> w1855 mode=indexing
                i -> [w1866]
                n1195 = Add(x=w1867, y=w1866) -> (x+y=w1865:i64)
              }
              n1196 = local write "Progress..."(u32 0 ("Progress...")) -> ()
              n1197 = local write "frames 2 play"(w1855) -> ()
            }
            frame #1 {
              w1872 = TRUE ("Play")
              w1873 = FALSE ("Next")
              n1198 = local write "Next"(w1873) -> ()
              n1199 = local write "Previous"(w1873) -> ()
              n1200 = local write "Reset"(w1873) -> ()
              n1201 = local write "stop"(w1873) -> ()
              n1202 = local write "Pause"(w1873) -> ()
              n1203 = local write "Load video"(w1872) -> ()
              n1204 = local write "Play"(w1872) -> ()
            }
          }
          n1205 = Index Array(array=w1841, index (col)=0 ("disabled index (col)")) -> (element=w1851:i64[])  [unwired: 1 in]
          n1206 = Search 1D Array(1D array=w1851, element=w1845) -> (index of element=w1850:i32)  [unwired: 1 in]
          n1207 = Index Array(array=w1841, index (row)=w1850) -> (element=w1849:i64[])  [unwired: 1 in]
          n1208 = Delete From Array(array=w1849, index=0) -> (array with subset deleted=w1848:i64[])  [unwired: 1 in, 1 out]
          n1209 = for {
            tunnel: w1848 -> [w1878] mode=indexing
            tunnel: [w1874] -> w1847 mode=indexing
            n1210 = Equal To 0?(x=w1878) -> (x = 0?=w1877:bool)
            n1211 = Select(t=FALSE ("x = 0?"), s=w1877, f=TRUE) -> (s? t:f=w1874:bool)
          }
          n1212 = Index Array(array=w1847) -> (element #1=w1838:bool, element #2=w1837:bool, element #3=w1836:bool, element #4=w1835:bool, element #5=w1834:bool, element #6=w1833:bool, element #7=w1832:bool, element #8=w1831:bool, element #9=w1830:bool, element #10=w1829:bool, element #11=w1828:bool, element #12=w1827:bool, element #13=w1826:bool, element #14=w1825:bool, element #15=w1824:bool, element #16=w1823:bool, element #17=w1822:bool, element #18=w1821:bool, element #19=w1820:bool, element #20=w1819:bool, element #21=w1818:bool, element #22=w1817:bool, element #23=w1816:bool, element #24=w1815:bool, element #25=w1814:bool, element #26=w1813:bool, element #27=w1812:bool, element #28=w1811:bool, element #29=w1810:bool, element #30=w1809:bool, element #31=w1808:bool, element #32=w1807:bool, element #33=w1806:bool, element #34=w1805:bool, element #35=w1802:bool, element #36=w1801:bool, element #39=w1800:bool, element #40=w1799:bool, element #41=w1798:bool, element #42=w1797:bool, element #43=w1796:bool, element #44=w1795:bool, element #45=w1794:bool, element #46=w1793:bool, element #47=w1792:bool, element #48=w1791:bool, element #49=w1790:bool, element #50=w1789:bool, element #51=w1788:bool, element #52=w1787:bool, element #53=w1786:bool)  [unwired: 53 in, 2 out]
          n1213 = Or(x=w1806, y=w1805) -> (x .or. y?=w1803:bool)
          n1214 = Or(x=w1808, y=w1807) -> (x .or. y?=w1804:bool)
          n1215 = local write "TL"(w1838) -> ()
          n1216 = local write "TCL"(w1837) -> ()
          n1217 = local write "TC"(w1836) -> ()
          n1218 = local write "TCR"(w1835) -> ()
          n1219 = local write "TR"(w1834) -> ()
          n1220 = local write "ML"(w1833) -> ()
          n1221 = local write "MCL"(w1832) -> ()
          n1222 = local write "MC"(w1831) -> ()
          n1223 = local write "MCR"(w1830) -> ()
          n1224 = local write "MR"(w1829) -> ()
          n1225 = local write "BL"(w1828) -> ()
          n1226 = local write "BCL"(w1827) -> ()
          n1227 = local write "BC"(w1826) -> ()
          n1228 = local write "BCR"(w1825) -> ()
          n1229 = local write "BR"(w1824) -> ()
          n1230 = local write "FH 2"(w1823) -> ()
          n1231 = local write "BH 2"(w1822) -> ()
          n1232 = local write "OH 2"(w1821) -> ()
          n1233 = local write "ST"(w1820) -> ()
          n1234 = local write "CR 2"(w1819) -> ()
          n1235 = local write "smash"(w1818) -> ()
          n1236 = local write "Dr def"(w1817) -> ()
          n1237 = local write "drive"(w1816) -> ()
          n1238 = local write "lob"(w1815) -> ()
          n1239 = local write "drop"(w1814) -> ()
          n1240 = local write "Hf smash"(w1813) -> ()
          n1241 = local write "clear"(w1812) -> ()
          n1242 = local write "net"(w1811) -> ()
          n1243 = local write "Blk def"(w1810) -> ()
          n1244 = local write "clear def"(w1809) -> ()
          n1245 = local write "winner"(w1804) -> ()
          n1246 = local write "error"(w1803) -> ()
          n1247 = local write "point 1"(w1802) -> ()
          n1248 = local write "point 2"(w1801) -> ()
          n1249 = local write "service1"(w1800) -> ()
          n1250 = local write "service2"(w1799) -> ()
          n1251 = local write "service3"(w1798) -> ()
          n1252 = local write "service4"(w1797) -> ()
          n1253 = local write "1 9"(w1796) -> ()
          n1254 = local write "2 9"(w1795) -> ()
          n1255 = local write "3 8"(w1794) -> ()
          n1256 = local write "4 8"(w1793) -> ()
          n1257 = local write "5 8"(w1792) -> ()
          n1258 = local write "Team 1"(w1791) -> ()
          n1259 = local write "Team 2"(w1790) -> ()
          n1260 = local write "player1"(w1789) -> ()
          n1261 = local write "player2"(w1788) -> ()
          n1262 = local write "player3"(w1787) -> ()
          n1263 = local write "player4"(w1786) -> ()
          n1264 = local read "refnum of data save file"() -> (w1839:refnum<file>)
        }
        frame "Edit coding" {
          n1265 = local read "Examine code"() -> (w1880:bool)
          n1266 = case shown="False" w1880 {
            tunnel: [T2."Edit video" ("Main tab") w1939] -> w1882
            frame False {
              n1267 = local read "Last Edit"() -> (w1898:bool[])
              n1268 = Index Array(array=w1898) -> (element #1=w1936:bool, element #2=w1935:bool, element #3=w1934:bool, element #4=w1933:bool, element #5=w1932:bool, element #6=w1931:bool, element #7=w1930:bool, element #8=w1929:bool, element #9=w1928:bool, element #10=w1927:bool, element #11=w1926:bool, element #12=w1925:bool, element #13=w1924:bool, element #14=w1923:bool, element #15=w1922:bool, element #16=w1921:bool, element #17=w1920:bool, element #18=w1919:bool, element #19=w1918:bool, element #20=w1917:bool, element #21=w1916:bool, element #22=w1915:bool, element #23=w1914:bool, element #24=w1913:bool, element #25=w1912:bool, element #26=w1911:bool, element #27=w1910:bool, element #28=w1909:bool, element #29=w1908:bool, element #30=w1907:bool, element #31=w1906:bool, element #32=w1905:bool, element #33=w1904:bool, element #34=w1903:bool, element #35=w1900:bool, element #36=w1899:bool, element #37=w1897:bool, element #38=w1896:bool, element #39=w1895:bool, element #40=w1894:bool, element #41=w1893:bool, element #42=w1892:bool, element #43=w1891:bool, element #44=w1890:bool, element #45=w1889:bool, element #46=w1888:bool, element #47=w1887:bool, element #48=w1886:bool, element #49=w1885:bool, element #50=w1884:bool, element #51=w1883:bool)  [unwired: 51 in]
              n1269 = Or(x=w1904, y=w1903) -> (x .or. y?=w1901:bool)
              n1270 = Or(x=w1906, y=w1905) -> (x .or. y?=w1902:bool)
              n1271 = local write "TL"(w1936) -> ()
              n1272 = local write "TCL"(w1935) -> ()
              n1273 = local write "TC"(w1934) -> ()
              n1274 = local write "TCR"(w1933) -> ()
              n1275 = local write "TR"(w1932) -> ()
              n1276 = local write "ML"(w1931) -> ()
              n1277 = local write "MCL"(w1930) -> ()
              n1278 = local write "MC"(w1929) -> ()
              n1279 = local write "MCR"(w1928) -> ()
              n1280 = local write "MR"(w1927) -> ()
              n1281 = local write "BL"(w1926) -> ()
              n1282 = local write "BCL"(w1925) -> ()
              n1283 = local write "BC"(w1924) -> ()
              n1284 = local write "BCR"(w1923) -> ()
              n1285 = local write "BR"(w1922) -> ()
              n1286 = local write "FH 2"(w1921) -> ()
              n1287 = local write "BH 2"(w1920) -> ()
              n1288 = local write "OH 2"(w1919) -> ()
              n1289 = local write "ST"(w1918) -> ()
              n1290 = local write "CR 2"(w1917) -> ()
              n1291 = local write "smash"(w1916) -> ()
              n1292 = local write "Dr def"(w1915) -> ()
              n1293 = local write "drive"(w1914) -> ()
              n1294 = local write "lob"(w1913) -> ()
              n1295 = local write "drop"(w1912) -> ()
              n1296 = local write "Hf smash"(w1911) -> ()
              n1297 = local write "clear"(w1910) -> ()
              n1298 = local write "net"(w1909) -> ()
              n1299 = local write "Blk def"(w1908) -> ()
              n1300 = local write "clear def"(w1907) -> ()
              n1301 = local write "winner"(w1902) -> ()
              n1302 = local write "error"(w1901) -> ()
              n1303 = local write "point 1"(w1900) -> ()
              n1304 = local write "point 2"(w1899) -> ()
              n1305 = local write "service1"(w1897) -> ()
              n1306 = local write "service2"(w1896) -> ()
              n1307 = local write "service3"(w1895) -> ()
              n1308 = local write "service4"(w1894) -> ()
              n1309 = local write "1 9"(w1893) -> ()
              n1310 = local write "2 9"(w1892) -> ()
              n1311 = local write "3 8"(w1891) -> ()
              n1312 = local write "4 8"(w1890) -> ()
              n1313 = local write "5 8"(w1889) -> ()
              n1314 = local write "Team 1"(w1888) -> ()
              n1315 = local write "Team 2"(w1887) -> ()
              n1316 = local write "player1"(w1886) -> ()
              n1317 = local write "player2"(w1885) -> ()
              n1318 = local write "player3"(w1884) -> ()
              n1319 = local write "player4"(w1883) -> ()
              n1320 = local write "Upload edited video"(TRUE ("Upload edited video")) -> ()
            }
            frame True {
              n1321 = case shown="True" "Next" {
                frame False {
                }
                frame True {
                  n1322 = local read "edited\nevents"() -> (w1953:i64[][])
                  n1323 = local read "Code number"() -> (w1957:i32)
                  n1324 = Increment(x=w1957) -> (x+1=w1951:i32)
                  n1325 = Index Array(array=w1953, index (col)=0 ("disabled index (col)")) -> (element=w1955:i64[])  [unwired: 1 in]
                  n1326 = Array Size(array=w1955) -> (size(s)=w1956:i32)
                  n1327 = Decrement(x=w1956) -> (x-1=w1950:i32)
                  n1328 = Less Or Equal?(x=w1951, y=w1950) -> (x <= y?=w1952:bool)
                  n1329 = Select(t=w1951, s=w1952, f=w1950) -> (s? t:f=w1949:i32)
                  n1330 = local write "Code number"(w1949) -> ()
                }
              }
              n1331 = case shown="True" "Previous" {
                frame False {
                }
                frame True {
                  n1332 = local read "Code number"() -> (w1962:i32)
                  n1333 = Decrement(x=w1962) -> (x-1=w1960:i32)
                  n1334 = Greater Or Equal To 0?(x=w1960) -> (x >= 0?=w1961:bool)
                  n1335 = Select(t=w1960, s=w1961, f=0) -> (s? t:f=w1958:i32)
                  n1336 = local write "Code number"(w1958) -> ()
                }
              }
              n1337 = Compound Arithmetic op=OR("Reset", "Previous", "Next") -> (w1945:bool)
              n1338 = Select(t=T2."Examine coding" ("Main tab"), s=w1945, f=T2."Edit coding" ("Main tab")) -> (s? t:f=w1940:T2)
              n1339 = Select(t=T2."Update coding" ("Main tab"), s="Update", f=w1940) -> (s? t:f=w1939:T2)
            }
          }
          n1340 = local read "refnum of data save file"() -> (w1879:refnum<file>)
        }
        frame "Update coding" {
          w1981 = "\r"
          n1341 = flat-sequence {
            tunnel: w1986 -> [w2058]
            tunnel: [w2055] -> w1985
            tunnel: w1985 -> [w2123]
            tunnel: [w2123] -> w1972
            frame #0 {
              w2037 = FALSE ("element")
              n1342 = local read "Team 1"() -> (w2019:bool)
              n1343 = local read "Team 2"() -> (w2023:bool)
              n1344 = local read "player1"() -> (w2020:bool)
              n1345 = local read "player2"() -> (w2021:bool)
              n1346 = local read "player3"() -> (w2022:bool)
              n1347 = local read "player4"() -> (w2024:bool)
              n1348 = local read "point 1"() -> (w2029:bool)
              n1349 = local read "point 2"() -> (w2030:bool)
              n1350 = local read "winner"() -> (w2025:bool)
              n1351 = local read "error"() -> (w2027:bool)
              n1352 = Compound Arithmetic op=OR(w2019, w2020, w2021) -> (w2026:bool)
              n1353 = Compound Arithmetic op=OR(w2023, w2022, w2024) -> (w2028:bool)
              n1354 = And(x=w2026, y=w2025) -> (x .and. y?=w2031:bool)
              n1355 = And(x=w2025, y=w2028) -> (x .and. y?=w2032:bool)
              n1356 = And(x=w2026, y=w2027) -> (x .and. y?=w2033:bool)
              n1357 = And(x=w2027, y=w2028) -> (x .and. y?=w2034:bool)
              n1358 = Compound Arithmetic op=OR(w2031, w2034, w2029) -> (w2035:bool)
              n1359 = Compound Arithmetic op=OR(w2033, w2032, w2030) -> (w2036:bool)
              n1360 = local read "Hf smash"() -> (w2014:bool)
              n1361 = local read "clear def"() -> (w2018:bool)
              n1362 = local read "Blk def"() -> (w2017:bool)
              n1363 = local read "smash"() -> (w2009:bool)
              n1364 = local read "Dr def"() -> (w2010:bool)
              n1365 = local read "OH 2"() -> (w2006:bool)
              n1366 = local read "MCR"() -> (w1997:bool)
              n1367 = local read "drive"() -> (w2011:bool)
              n1368 = local read "MCL"() -> (w1995:bool)
              n1369 = local read "BH 2"() -> (w2005:bool)
              n1370 = local read "drop"() -> (w2013:bool)
              n1371 = local read "clear"() -> (w2015:bool)
              n1372 = local read "FH 2"() -> (w2004:bool)
              n1373 = local read "CR 2"() -> (w2008:bool)
              n1374 = local read "TCR"() -> (w1992:bool)
              n1375 = local read "BCR"() -> (w2002:bool)
              n1376 = local read "TCL"() -> (w1990:bool)
              n1377 = local read "BCL"() -> (w2000:bool)
              n1378 = local read "MC"() -> (w1996:bool)
              n1379 = local read "MR"() -> (w1998:bool)
              n1380 = local read "service1"() -> (w2038:bool)
              n1381 = local read "service2"() -> (w2039:bool)
              n1382 = local read "service3"() -> (w2040:bool)
              n1383 = local read "service4"() -> (w2041:bool)
              n1384 = local read "ML"() -> (w1994:bool)
              n1385 = local read "lob"() -> (w2012:bool)
              n1386 = local read "net"() -> (w2016:bool)
              n1387 = local read "TC"() -> (w1991:bool)
              n1388 = local read "BC"() -> (w2001:bool)
              n1389 = local read "Team 1"() -> (w2047:bool)
              n1390 = local read "Team 2"() -> (w2048:bool)
              n1391 = local read "TR"() -> (w1993:bool)
              n1392 = local read "BR"() -> (w2003:bool)
              n1393 = local read "player1"() -> (w2051:bool)
              n1394 = local read "player2"() -> (w2052:bool)
              n1395 = local read "player3"() -> (w2053:bool)
              n1396 = local read "player4"() -> (w2054:bool)
              n1397 = local read "TL"() -> (w1989:bool)
              n1398 = local read "BL"() -> (w1999:bool)
              n1399 = local read "ST"() -> (w2007:bool)
              n1400 = local read "1 9"() -> (w2042:bool)
              n1401 = local read "2 9"() -> (w2043:bool)
              n1402 = local read "3 8"() -> (w2044:bool)
              n1403 = local read "4 8"() -> (w2045:bool)
              n1404 = local read "5 8"() -> (w2046:bool)
              n1405 = Compound Arithmetic op=OR(w2047, w2051, w2052) -> (w2049:bool)
              n1406 = Compound Arithmetic op=OR(w2048, w2053, w2054) -> (w2050:bool)
              n1407 = Build Array(w1989, w1990, w1991, w1992, w1993, w1994, w1995, w1996, w1997, w1998, w1999, w2000, w2001, w2002, w2003, w2004, w2005, w2006, w2007, w2008, w2009, w2010, w2011, w2012, w2013, w2014, w2015, w2016, w2017, w2018, w2031, w2032, w2033, w2034, w2035, w2036, w2037, w2037, w2038, w2039, w2040, w2041, w2042, w2043, w2044, w2045, w2046, w2049, w2050, w2051, w2052, w2053, w2054) -> (w1988:bool[])
              n1408 = Boolean To (0,1)(Boolean=w1988) -> (0, 1=w2060:i16[])
              n1409 = local read "Code number"() -> (w2068:i32)
              n1410 = local read "edited\nevents"() -> (w2061:i64[][])
              n1411 = Index Array(array=w2061, index (row)=w2068, index (col)=0) -> (element=w2063:i64)
              n1412 = Index Array(array=w2058, index (col)=0 ("disabled index (col)")) -> (element=w2065:i64[])  [unwired: 1 in]
              n1413 = Search 1D Array(1D array=w2065, element=w2063) -> (index of element=w2056:i32)  [unwired: 1 in]
              n1414 = Index Array(array=w2058, index (row)=w2056) -> (element=w2064:i64[])  [unwired: 1 in]
              n1415 = Delete From Array(array=w2064, index=0) -> (deleted portion=w2059:i64)  [unwired: 1 in, 1 out]
              n1416 = Build Array (concatenate)(w2059, w2060) -> (w2057:i64[])
              n1417 = Replace Array Subset(array=w2058, new element=w2057, index (row)=w2056) -> (w2055:i64[][])  [unwired: 1 in]
            }
            frame #1 {
              n1418 = local read "Last Edit"() -> (w2084:bool[])
              n1419 = Index Array(array=w2084) -> (element #1=w2122:bool, element #2=w2121:bool, element #3=w2120:bool, element #4=w2119:bool, element #5=w2118:bool, element #6=w2117:bool, element #7=w2116:bool, element #8=w2115:bool, element #9=w2114:bool, element #10=w2113:bool, element #11=w2112:bool, element #12=w2111:bool, element #13=w2110:bool, element #14=w2109:bool, element #15=w2108:bool, element #16=w2107:bool, element #17=w2106:bool, element #18=w2105:bool, element #19=w2104:bool, element #20=w2103:bool, element #21=w2102:bool, element #22=w2101:bool, element #23=w2100:bool, element #24=w2099:bool, element #25=w2098:bool, element #26=w2097:bool, element #27=w2096:bool, element #28=w2095:bool, element #29=w2094:bool, element #30=w2093:bool, element #31=w2092:bool, element #32=w2091:bool, element #33=w2090:bool, element #34=w2089:bool, element #35=w2086:bool, element #36=w2085:bool, element #37=w2083:bool, element #38=w2082:bool, element #39=w2081:bool, element #40=w2080:bool, element #41=w2079:bool, element #42=w2078:bool, element #43=w2077:bool, element #44=w2076:bool, element #45=w2075:bool, element #46=w2074:bool, element #47=w2073:bool, element #48=w2072:bool, element #49=w2071:bool, element #50=w2070:bool, element #51=w2069:bool)  [unwired: 51 in]
              n1420 = Or(x=w2090, y=w2089) -> (x .or. y?=w2087:bool)
              n1421 = Or(x=w2092, y=w2091) -> (x .or. y?=w2088:bool)
              n1422 = local write "TL"(w2122) -> ()
              n1423 = local write "TCL"(w2121) -> ()
              n1424 = local write "TC"(w2120) -> ()
              n1425 = local write "TCR"(w2119) -> ()
              n1426 = local write "TR"(w2118) -> ()
              n1427 = local write "ML"(w2117) -> ()
              n1428 = local write "MCL"(w2116) -> ()
              n1429 = local write "MC"(w2115) -> ()
              n1430 = local write "MCR"(w2114) -> ()
              n1431 = local write "MR"(w2113) -> ()
              n1432 = local write "BL"(w2112) -> ()
              n1433 = local write "BCL"(w2111) -> ()
              n1434 = local write "BC"(w2110) -> ()
              n1435 = local write "BCR"(w2109) -> ()
              n1436 = local write "BR"(w2108) -> ()
              n1437 = local write "FH 2"(w2107) -> ()
              n1438 = local write "BH 2"(w2106) -> ()
              n1439 = local write "OH 2"(w2105) -> ()
              n1440 = local write "ST"(w2104) -> ()
              n1441 = local write "CR 2"(w2103) -> ()
              n1442 = local write "smash"(w2102) -> ()
              n1443 = local write "Dr def"(w2101) -> ()
              n1444 = local write "drive"(w2100) -> ()
              n1445 = local write "lob"(w2099) -> ()
              n1446 = local write "drop"(w2098) -> ()
              n1447 = local write "Hf smash"(w2097) -> ()
              n1448 = local write "clear"(w2096) -> ()
              n1449 = local write "net"(w2095) -> ()
              n1450 = local write "Blk def"(w2094) -> ()
              n1451 = local write "clear def"(w2093) -> ()
              n1452 = local write "winner"(w2088) -> ()
              n1453 = local write "error"(w2087) -> ()
              n1454 = local write "point 1"(w2086) -> ()
              n1455 = local write "point 2"(w2085) -> ()
              n1456 = local write "service1"(w2083) -> ()
              n1457 = local write "service2"(w2082) -> ()
              n1458 = local write "service3"(w2081) -> ()
              n1459 = local write "service4"(w2080) -> ()
              n1460 = local write "1 9"(w2079) -> ()
              n1461 = local write "2 9"(w2078) -> ()
              n1462 = local write "3 8"(w2077) -> ()
              n1463 = local write "4 8"(w2076) -> ()
              n1464 = local write "5 8"(w2075) -> ()
              n1465 = local write "Team 1"(w2074) -> ()
              n1466 = local write "Team 2"(w2073) -> ()
              n1467 = local write "player1"(w2072) -> ()
              n1468 = local write "player2"(w2071) -> ()
              n1469 = local write "player3"(w2070) -> ()
              n1470 = local write "player4"(w2069) -> ()
            }
          }
          n1471 = local read "Name 1"() -> (w1964:string)
          n1472 = local read "Name 2"() -> (w1965:string)
          n1473 = local read "Name 3"() -> (w1966:string)
          n1474 = local read "Name 4"() -> (w1967:string)
          n1475 = Build Array(w1964, w1965, w1966, w1967) -> (w1963:string[])
          n1476 = call "EVENTS(SubVI).vi"() -> ("Events"=w1969:string)  [unwired: 1 in]
          n1477 = local read "Video file"() -> (w1978:path)
          n1478 = call "Doubles Events (SubVI).vi"("Singles Events"=w1969, "PLAYER NAMES"=w1963) -> ("Edited Events For Doubles"=w1968:string)
          n1479 = local read "Data file"() -> (w1971:path)
          n1480 = call <vilib>:"Get File Extension.vi"("file"=w1978) -> ("filename without extension"=w1980:string)  [unwired: 7 in, 3 out]
          n1481 = Array To Spreadsheet String(delimiter (Tab)="\t" ("delimiter (\\t)"), array=w1972, 3:"%.3f" ("format (%.3f)")) -> (spreadsheet string=w1983:string)
          n1482 = Open/Create/Replace File(file path (use dialog)=w1971, operation (0:open)=T3."replace") -> (refnum out=w1974:refnum<file>, error out=w1973:errorcluster)  [unwired: 4 in, 1 out]
          n1483 = Concatenate Strings("avi file" ("string"), w1981, w1980, w1981, w1981, w1968, w1983) -> (w1982:string)
          n1484 = Write to Text File(file (use dialog)=w1974, text=w1982, error in=w1973) -> (refnum out=w1970:refnum<file>)  [unwired: 1 in, 2 out]
          n1485 = local write "Update"(FALSE ("Update")) -> ()
        }
      }
      "refnum of data save file" <- w370
      n1486 = Equal?(x="Main tab", y=enum32{"Coding", "Display"}."Coding" ("Tab Control 3")) -> (x = y?=w382:bool)
      n1487 = Not Equal?(x=w376, y=w375) -> (x != y?=w381:bool)
      n1488 = Select(t=w375, s=w382, f=w378) -> (s? t:f=w379:T2)
      n1489 = And(x=w381, y=w382) -> (x .and. y?=w380:bool)
      n1490 = Equal?(x=w376, y=w375) -> (x = y?=w374:bool)
      n1491 = Equal?(x=w379, y=w378) -> (x = y?=w377:bool)
      n1492 = And(x=w377, y=w374) -> (x .and. y?=w373:bool)
      n1493 = case shown="True" w380 {
        tunnel: w372 -> [_ w391]
        frame False {
        }
        frame True {
          # "Moving back to coding tab"
          n1494 = flat-sequence {
            tunnel: w391 -> [w395]
            frame #0 {
              n1495 = local read "ful video frames"() -> (w396:i64[])
              n1496 = Index Array(array=w395, index (col)=0 ("disabled index (col)")) -> (element=w393:i64[])  [unwired: 1 in]
              n1497 = Array Max & Min(array=w393) -> (max value=w392:i64)  [unwired: 3 out]
              n1498 = local write "frames 2 play"(w396) -> ()
              n1499 = local write "Progress..."(w392) -> ()
            }
            frame #1 {
              w397 = FALSE ("Next")
              w398 = TRUE ("Play")
              n1500 = local write "stop"(w398) -> ()
              n1501 = local write "Load video"(w398) -> ()
              n1502 = local write "Pause"(w397) -> ()
              n1503 = local write "Update"(w397) -> ()
              n1504 = local write "Next"(w397) -> ()
              n1505 = local write "Previous"(w397) -> ()
              n1506 = local write "Reset"(w397) -> ()
              n1507 = local write "Extract data"(w397) -> ()
              n1508 = local write "Upload edited video"(w397) -> ()
              n1509 = local write "Examine code"(w397) -> ()
            }
          }
        }
      }
      n1510 = case shown="True" w373 {
        frame False {
        }
        frame True {
          n1511 = local write "Progress..."(u32 0 ("Progress...")) -> ()
          n1512 = local write "Pause"(FALSE ("Pause")) -> ()
          n1513 = local write "stop"(TRUE ("stop")) -> ()
        }
      }
      n1514 = local read "START"() -> (w371:bool)
      n1515 = Wait (ms)(milliseconds to wait=u32 200) -> ()  [unwired: 1 out]
    }
    n1516 = while {
      tunnel: w10 -> [w221]
      tunnel: w1 -> [_]
      tunnel: [w216] -> w5
      stop <- w216 continue-if-true
      # "This loop is for writing\nvideo to disk"
      n1517 = local read "Video files to write"() -> (w220:string[])
      n1518 = local read "frames to write"() -> (w218:i64[][])
      n1519 = case shown="True" "Write file" {
        tunnel: [FALSE FALSE] -> w223
        tunnel: w221 -> [_ w241]
        tunnel: w220 -> [_ w240]
        tunnel: "Video to write" -> [_ w239]
        tunnel: w218 -> [_ w238]
        tunnel: [u32 0 ("milliseconds to wait") u32 0 ("milliseconds to wait")] -> w217
        frame False {
          w225 = T4."Enabled" ("Disabled")
          n1520 = local read "Video files to write"() -> (w229:string[])
          n1521 = property on="Add to lib" class="Bool (strict)"("DisabledEnum"=w225) -> ()  [unwired: 2 in, 2 out]
          n1522 = property on="File name" class="Str"("DisabledEnum"=w225) -> ()  [unwired: 2 in, 2 out]
          n1523 = property on="Video to write" class="Path"("DisabledEnum"=w225) -> ()  [unwired: 2 in, 2 out]
          n1524 = property on="START" class="Bool (strict)"("DisabledEnum"=w225) -> ()  [unwired: 2 in, 2 out]
          n1525 = Empty Array?(array=w229) -> (empty?=w228:bool)
          n1526 = Select(t=T4."Disabled and Grayed Out" ("Disabled"), s=w228, f=w225) -> (s? t:f=w226:T4)
          n1527 = property on="Write file" class="Bool (strict)"("DisabledEnum"=w226) -> ()  [unwired: 2 in, 2 out]
          n1528 = local write "Abort"(FALSE ("Abort")) -> ()
        }
        frame True {
          w233 = T4."Disabled and Grayed Out" ("Disabled")
          n1529 = for {
            tunnel: w238 -> [w280] mode=indexing
            tunnel: w240 -> [w271] mode=indexing
            tunnel: w239 -> [w270]
            tunnel: w241 -> [w258]
            tunnel: [w252] -> w236
            tunnel: [w251] -> w235
            tunnel: [w249] -> w234
            i -> [w253]
            stop <- w250 stop-if-true
            w267 = T5 4 items=["Grayscale (U8)", "Grayscale (I16)", "Grayscale (SGL)", "Complex (CSG)", "RGB (U32)", "HSL (U32)", "RGB (U64)"] ("Image Type")
            n1530 = Path To String(path=w270) -> (string=w272:string)
            n1531 = for {
              tunnel: w280 -> [w318] mode=indexing
              tunnel: [w318] -> w257 mode=indexing if=w317
              n1532 = Not Equal To 0?(x=w318) -> (x != 0?=w317:bool)
            }
            n1533 = Concatenate Strings(w272, "\\" ("string"), w271) -> (w275:string)
            n1534 = Array Size(array=w257) -> (size(s)=w256:i32)
            n1535 = Decrement(x=w253) -> (x-1=w254:i32)
            n1536 = Not Equal To 0?(x=w253) -> (x != 0?=w255:bool)
            n1537 = call <vilib>:"Search and Replace Pattern.vi"("string"=w275, "regular expression (\"\")"=".avi" ("regular expression (\"\")")) -> ("result string"=w279:string)  [unwired: 3 in, 1 out]
            n1538 = case shown="True" w255 {
              tunnel: w254 -> [_ w290]
              frame False {
              }
              frame True {
                n1539 = local read "Video files to write"() -> (w294:string[])
                n1540 = local read "frames to write"() -> (w291:i64[][])
                n1541 = Delete From Array(array=w294, index=w290) -> (array with subset deleted=w293:string[])  [unwired: 1 in, 1 out]
                n1542 = Delete From Array(array=w291, index (row)=w290) -> (array with subset deleted=w292:i64[][])  [unwired: 2 in, 1 out]
                n1543 = local write "frames to write"(w292) -> ()
                n1544 = local write "Video files to write"(w293) -> ()
              }
            }
            n1545 = property on="Writing" class="Slide (strict)"("Scale.Maximum"=w256) -> ()  [unwired: 2 in, 2 out]
            n1546 = Concatenate Strings(w279, ".avi" ("string")) -> (w277:string)
            n1547 = String To Path(string=w277) -> (path=w278:path)
            n1548 = while {
              shift-right: [w298] -> _
              shift-left: w278 -> [w297]
              tunnel: w279 -> [w302]
              tunnel: [w297] -> w248
              i -> [w296]
              stop <- w304 continue-if-true
              n1549 = Increment(x=w296) -> (x+1=w295:i32)
              n1550 = call <vilib>:"Check if File or Folder Exists.vi"("path"=w297) -> ("file or folder exists?"=w304:bool)  [unwired: 8 in, 2 out]
              n1551 = Number To Decimal String(number=w295) -> (decimal integer string=w301:string)  [unwired: 1 in]
              n1552 = Concatenate Strings(w302, " (file path clash) - " ("string"), w301, ".avi" ("string")) -> (w299:string)
              n1553 = String To Path(string=w299) -> (path=w298:path)
            }
            n1554 = Select(t="Microsoft Video 1" ("Codec Name"), s="Video compress", f="" ("Codec Name")) -> (s? t:f=w244:string)
            n1555 = local read "framesPerSecond"() -> (w261:u32)
            n1556 = call "IMAQ AVI Create"("Compression Filter"=w244, "Frames Per Second"=w261, "AVI Path"=w248) -> ("error out"=w268:errorcluster, "Avi Refnum"=w262:T6)  [unwired: 7 in]
            n1557 = call "IMAQ Create"("Image Name"="write", "Image Type"=w267, "error in (no error)"=w268) -> ("New Image"=w266:T1, "error out"=w265:errorcluster)  [unwired: 2 in]
            n1558 = for {
              tunnel: w257 -> [w315] mode=indexing
              tunnel: w266 -> [w309]
              tunnel: w265 -> [w314]
              tunnel: [w312] -> w264
              tunnel: [w311] -> w263
              tunnel: w262 -> [w310]
              tunnel: [w309] -> w259
              tunnel: w258 -> [w308]
              tunnel: ["Abort"] -> w250
              i -> [w307]
              stop <- "Abort" stop-if-true
              n1559 = Increment(x=w307) -> (x+1=→"Writing":i32)
              n1560 = call "IMAQ AVI Read Frame"("error in (no error)"=w314, "Frame Number"=w315, "Image"=w309, "Avi Refnum"=w308) -> ("error out"=w316:errorcluster, "Image Out"=w313:T1)  [unwired: 4 in, 2 out]
              n1561 = call "IMAQ AVI Write Frame"("error in (no error)"=w316, "Image"=w313, "Avi Refnum"=w310) -> ("error out"=w311:errorcluster, "Avi Refnum (duplicate)"=w312:T6)  [unwired: 7 in]
            }
            n1562 = call "IMAQ AVI Close"("error in (no error)"=w263, "Avi Refnum"=w264) -> ("error out"=w260:errorcluster)  [unwired: 9 in]
            n1563 = call "IMAQ Dispose"("Image"=w259, "error in (no error)"=w260) -> ("error out"=w247:errorcluster)  [unwired: 4 in]
            n1564 = case shown="False" w250 {
              tunnel: [string[] [] ("Video files to write") w288] -> w252
              tunnel: [i64[][] [] ("to write") w287] -> w251
              tunnel: ["Writing Complete" ("message") "Writing aborted" ("message")] -> w249
              tunnel: w248 -> [_ w285]
              tunnel: w247 -> [_ w284]
              frame False {
              }
              frame True {
                n1565 = local read "Video files to write"() -> (w288:string[])
                n1566 = Delete(path (use dialog)=w285, error in=w284) -> ()  [unwired: 3 in, 3 out]
                n1567 = local read "frames to write"() -> (w287:i64[][])
                n1568 = local write "Abort"(FALSE ("Abort")) -> ()
              }
            }
          }
          n1569 = One Button Dialog(message=w234) -> ()  [unwired: 1 in, 1 out]
          n1570 = local write "Video files to write"(w236) -> ()
          n1571 = local write "frames to write"(w235) -> ()
          n1572 = property on="Add to lib" class="Bool (strict)"("DisabledEnum"=w233) -> ()  [unwired: 2 in, 2 out]
          n1573 = property on="File name" class="Str"("DisabledEnum"=w233) -> ()  [unwired: 2 in, 2 out]
          n1574 = property on="Video to write" class="Path"("DisabledEnum"=w233) -> ()  [unwired: 2 in, 2 out]
          n1575 = property on="START" class="Bool (strict)"("DisabledEnum"=w233) -> ()  [unwired: 2 in, 2 out]
        }
      }
      n1576 = local read "START"() -> (w216:bool)
      n1577 = local write "Write file"(w223) -> ()
      n1578 = local write "Writing"(w217) -> ()
      n1579 = Wait (ms)(milliseconds to wait=u32 200) -> ()  [unwired: 1 out]
    }
    n1580 = while {
      tunnel: [w182] -> w6
      tunnel: w1 -> [_]
      stop <- w182 continue-if-true
      n1581 = case shown="True" "REPORT" {
        frame False {
        }
        frame True {
          w206 = TRUE ("open new instance (false)")
          n1582 = local read "Data file"() -> (w192:path)
          n1583 = local read "Video file"() -> (w191:path)
          n1584 = local write "REPORT"(FALSE ("REPORT")) -> ()
          n1585 = Strip Path(path=w192) -> (stripped path=w190:path)  [unwired: 1 out]
          n1586 = call <vilib>:"Get File Extension.vi"("file"=w191) -> ("filename without extension"=w187:string)  [unwired: 7 in, 3 out]
          n1587 = Path To String(path=w190) -> (string=w189:string)
          n1588 = Concatenate Strings(w189, "\\" ("string"), w187, " (BStAT Report).doc" ("string")) -> (w193:string)
          n1589 = String To Path(string=w193) -> (path=w195:path)
          n1590 = call <vilib>:"Check if File or Folder Exists.vi"("path"=w195) -> ("file or folder exists?"=w194:bool)  [unwired: 8 in, 2 out]
          n1591 = Automation Open(Automation Refnum=refnum<k7> refnum ("Word._Application"), 9:w206) -> (Automation Refnum=w199:refnum<k7>, error out=w200:errorcluster)  [unwired: 2 in]
          n1592 = property class="_Application"(reference=w199, error in=w200, "Visible"=w206) -> (reference out=w201:refnum<k7>, error out=w202:errorcluster)
          n1593 = case shown="True" w194 {
            tunnel: w195 -> [w209 w215]
            tunnel: [w208 w215] -> w185
            frame False {
              n1594 = Current VI's Path() -> (path=w212:path)
              n1595 = Strip Path(path=w212) -> (stripped path=w211:path)  [unwired: 1 out]
              n1596 = Build Path(base path=w211, name or relative path="BStAT report.doc") -> (appended path=w210:path)
              n1597 = One Button Dialog(message="***New report generated***\n\nRight-click on the white strip on the LEFT of the data area to copy the data ") -> ()  [unwired: 1 in, 1 out]
              n1598 = Copy(10:w209, 11:w210) -> (3:w208:path)  [unwired: 3 in, 2 out]
            }
            frame True {
              n1599 = One Button Dialog(message="***Report found***\n\nRight-click on the white strip on the LEFT of the data area to copy the data ") -> ()  [unwired: 1 in, 1 out]
            }
          }
          n1600 = property class="_Application"(reference=w201, error in=w202) -> (error out=w204:errorcluster, "Documents"=w203:refnum<k7>)  [unwired: 1 out]
          n1601 = invoke class="Documents" method="Open"(reference=w203, error in=w204, "FileName"=w185, "ReadOnly"=TRUE, "Visible"=TRUE) -> ()  [unwired: 14 in, 19 out]
        }
      }
      n1602 = local read "START"() -> (w182:bool)
      n1603 = Wait (ms)(milliseconds to wait=u32 200) -> ()  [unwired: 1 out]
    }
    n1604 = flat-sequence {
      tunnel: w7 -> [w33]
      tunnel: w6 -> [_]
      tunnel: w5 -> [_]
      tunnel: w4 -> [w34]
      frame #0 {
        w28 = T5 4 items=["Grayscale (U8)", "Grayscale (I16)", "Grayscale (SGL)", "Complex (CSG)", "RGB (U32)", "HSL (U32)", "RGB (U64)"] ("Image Type")
        w29 = T5 4 items=["Grayscale (U8)", "Grayscale (I16)", "Grayscale (SGL)", "Complex (CSG)", "RGB (U32)", "HSL (U32)", "RGB (U64)"] ("Image Type")
        w31 = T5 4 items=["Grayscale (U8)", "Grayscale (I16)", "Grayscale (SGL)", "Complex (CSG)", "RGB (U32)", "HSL (U32)", "RGB (U64)"] ("Image Type")
        n1605 = call "IMAQ AVI Close"("Avi Refnum"=w34) -> ("error out"=w32:errorcluster)  [unwired: 10 in]
        n1606 = Close File(refnum=w33, error in=w32) -> (error out=w26:errorcluster)  [unwired: 1 out]
        n1607 = call "IMAQ Create"("Image Name"="Video", "Image Type"=w28, "error in (no error)"=w26) -> ("New Image"=w22:T1, "error out"=w25:errorcluster)  [unwired: 2 in]
        n1608 = call "IMAQ Create"("Image Name"="pauselag", "Image Type"=w31, "error in (no error)"=w25) -> ("New Image"=w21:T1, "error out"=w23:errorcluster)  [unwired: 2 in]
        n1609 = call "IMAQ Create"("Image Name"="write", "Image Type"=w29, "error in (no error)"=w23) -> ("New Image"=w20:T1, "error out"=w19:errorcluster)  [unwired: 2 in]
        n1610 = call "IMAQ Dispose"("Image"=w22, "error in (no error)"=w19) -> ("error out"=w18:errorcluster)  [unwired: 4 in]
        n1611 = call "IMAQ Dispose"("Image"=w21, "error in (no error)"=w18) -> ("error out"=w17:errorcluster)  [unwired: 4 in]
        n1612 = call "IMAQ Dispose"("Image"=w20, "error in (no error)"=w17) -> ()  [unwired: 4 in, 1 out]
      }
    }
    n1613 = Wait (ms)(milliseconds to wait=u32 100) -> ()  [unwired: 1 out]
  }
